vi "main.vi"() -> ()   [LabVIEW 2021]
uses:
  <vilib>/xnet/xnet.llb/XNET Frame CAN.ctl
  <vilib>/xnet/xnet.llb/XNET Frame Type CAN.ctl
  General Purpose/measurements.ctl
  General Purpose/measurements_SC.ctl
  active-front-ends/Time-sync/time_sync/TypeDef/Synch_shift--cluster.ctl
  <vilib>/Platform/TimedLoop/XDataNode/timing_clust.ctl
  <vilib>/Platform/TimedLoop/XDataNode/nitl_modes.ctl
  <vilib>/Platform/TimedLoop/XDataNode/wakeup.ctl
  communication/PVemulator_Central.ctl
  communication/PVemulator_Central_Info.ctl
  communication/PVemulator_Central_Data.ctl
  communication/SC_references.ctl
  central data acquisition/MeteoBoxCentral.ctl
  central data acquisition/MeteoBoxCentral_Info.ctl
  central data acquisition/MeteoBoxCentral_Data.ctl
  <vilib>/xnet/xnet.llb/XNET Write (Frame CAN).vi
  <vilib>/xnet/xnet.llb/XNET Read (Frame CAN).vi
  <vilib>/Platform/TimedLoop/XDataNode/XDataNode.xnode
  <vilib>/Platform/TimedLoop/XDataNode/XDNodeRunTimeDep.lvlib
  <userlib>/_OpenG.lib/boolean/boolean.llb/openg_boolean__ogtk.lvlib
panel:
  out "Period":i64
  out "follow":timestamp
  out "form":timestamp
  out "time_sc":timestamp
  out "start following SC pre":bool
  out "forming?":bool
  out "Ready SC":bool
  out "OFF SC":bool
  out "V slider 31":dbl(slide) caption="V-i" max=-10.0 scale=0.0..100.0 scale format="%#_4g"
  in  "SEND sp SC":bool
  in  "Start following SC":bool
  in  "Start forming SC":bool
  in  "Vdc SC":dbl
  out "Synch Monitor":string[][](table)
  in  "Loop Time":u32=125
  out "Error out":errorcluster
  in  "Timeout [ms]":i32=3000
  out "Offset from TR (ns)":dbl
  out "Status Out":T1
  out "ON SC":bool
  out "state SC":u16
  out "measurements SuperCap":T2
  out "V slider 29":dbl(slide) caption="V-i" max=-10.0 scale=650.0..780.0 scale format="%#_4g"
  out "V slider 30":dbl(slide) caption="V-i" max=-10.0 scale=650.0..780.0 scale format="%#_4g"
  out "kW":dbl caption="Numeric" format="%#.3g"
  in  "Pdc SC":dbl
  in  "Shutdwn SC":bool
  in  "Use METEO":bool
  out "Temps":dbl[](array[numeric])
  out "GHIs":dbl[](array[numeric])
  out "Meteo.Tair":dbl
  out "Meteo.GHI":dbl
  in  "Update setpoints":bool
  out "V slider 28":dbl(slide) caption="V-i" max=-10.0 scale=650.0..780.0 scale format="%#_4g"
  out "V slider 27":dbl(slide) caption="V-i" max=-10.0 scale=650.0..780.0 scale format="%#_4g"
  out "V slider 26":dbl(slide) caption="V-i" max=-10.0 scale=650.0..780.0 scale format="%#_4g"
  out "V slider 25":dbl(slide) caption="V-i" max=-10.0 scale=650.0..780.0 scale format="%#_4g"
  out "V slider 24":dbl(slide) caption="V-i" max=-10.0 scale=650.0..780.0 scale format="%#_4g"
  out "V slider 23":dbl(slide) caption="V-i" max=-10.0 scale=650.0..780.0 scale format="%#_4g"
  out "V slider 22":dbl(slide) caption="V-i" max=-10.0 scale=650.0..780.0 scale format="%#_4g"
  out "V slider 21":dbl(slide) caption="V-i" max=-10.0 scale=650.0..780.0 scale format="%#_4g"
  in  "P 4":dbl
  in  "P 3":dbl
  in  "P 2":dbl
  out "state 4":u16
  out "state 3":u16
  out "state 2":u16
  out "state 1":u16
  out "kW":dbl caption="Numeric" format="%#.3g"
  out "kW":dbl caption="Numeric" format="%#.3g"
  out "kW":dbl caption="Numeric" format="%#.3g"
  out "kW":dbl caption="Numeric" format="%#.3g"
  in  "P 1":dbl
  out "current time":timestamp
  in  "measurements":T3
  out "CAN OUT":T4 {"payload" format="%x"; "timestamp" format="%<%.7X\n%x>T"; "type" items=["CAN Data"=0, "CAN Remote"=1, "CAN Bus Error"=2, "CAN 2.0 Data"=8, "CAN FD Data"=16, "CAN FD+BRS Data"=24, "J1939 Data"=192, "Delay"=224, "Log Trigger"=225, "Start Trigger"=226]; "identifier" format="%x"}
  in  "EnablePR 4":bool
  in  "EnablePR 3":bool
  in  "EnablePR 2":bool
  in  "EnablePR 1":bool
  in  "main stop":bool
  in  "DCLinkOK  4":bool
  in  "PowerEnable 4":bool
  in  "ErrAck 4":bool
  in  "Shutdwn 4":bool
  in  "DCLinkOK  3":bool
  in  "PowerEnable 3":bool
  in  "ErrAck 3":bool
  in  "Shutdwn 3":bool
  in  "DCLinkOK 2":bool
  in  "PowerEnable 2":bool
  in  "ErrAck 2":bool
  in  "Shutdwn 2":bool
  out "OFF 4":bool
  out "ON 4":bool
  out "Ready 4":bool
  out "OFF 3":bool
  out "ON 3":bool
  out "Ready 3":bool
  out "OFF 2":bool
  out "ON 2":bool
  out "Ready 2":bool
  out "error out":errorcluster
  out "OFF 1":bool
  out "ON 1":bool
  out "Ready 1":bool
  out "CAN IN":T4 {"payload" format="%x"; "timestamp" format="%<%.7X\n%x>T"; "type" items=["CAN Data"=0, "CAN Remote"=1, "CAN Bus Error"=2, "CAN 2.0 Data"=8, "CAN FD Data"=16, "CAN FD+BRS Data"=24, "J1939 Data"=192, "Delay"=224, "Log Trigger"=225, "Start Trigger"=226]; "identifier" format="%x"}
  in  "CAN [ms]":i64=1
  out "CAN with Conv":bool
  out "Measurements":bool
  in  "Shutdwn 1":bool
  in  "ErrAck 1":bool
  in  "PowerEnable 1":bool
  in  "DCLinkOK 1":bool
  # "PV emulators 1-4"
  # "B22"
  # "DC"
  # "PV 4"
  # "DC"
  # "B21"
  # "DC"
  # "PV 3"
  # "DC"
  # "B20"
  # "DC"
  # "PV 2"
  # "DC"
  # "B19"
  # "1"
  # "DC"
  # "2"
  # "PV 1"
  # "3"
  # "DC"
  # "DC"
  # "SC"
  # "DC"
  # "SOC"
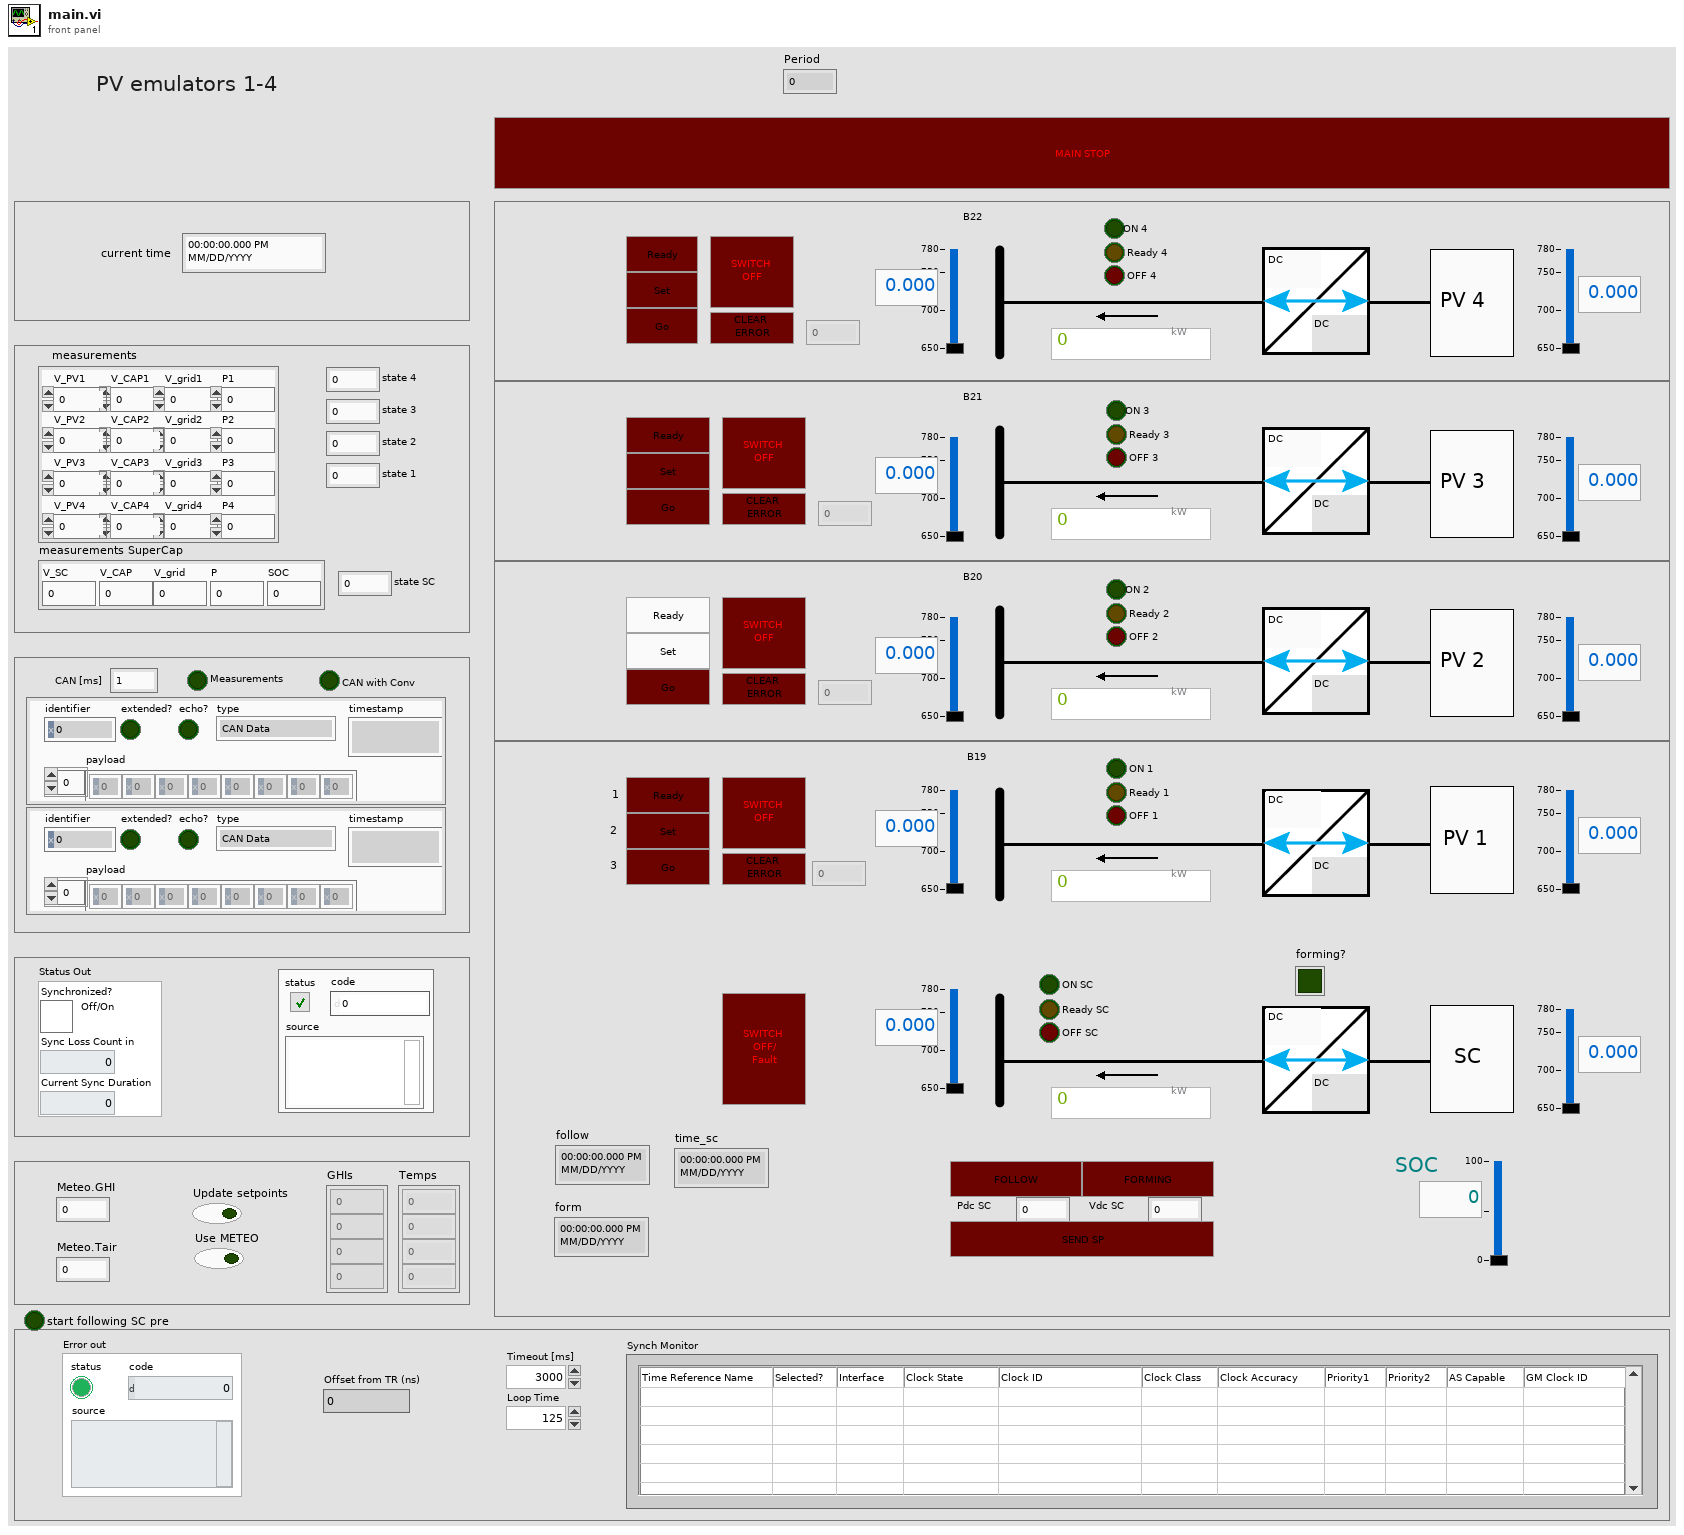
[diagram p1: front panel]
types:
  T1 = typedef "Synch_shift--cluster.ctl" = cluster{"Synchronized?":bool, "Sync Loss Count in":u32, "Current Sync Duration":u32}
  T2 = typedef "measurements_SC.ctl" = cluster{"V_SC":dbl, "V_CAP":dbl, "V_grid":dbl, "P":dbl, "SOC":dbl}
  T3 = typedef "measurements.ctl" = cluster{"V_PV1":dbl, "V_CAP1":dbl, "V_PV2":dbl, "V_CAP2":dbl, "V_grid2":dbl, "V_PV3":dbl, "V_CAP3":dbl, "V_grid3":dbl, "V_PV4":dbl, "V_CAP4":dbl, "V_grid4":dbl, "V_grid1":dbl, "P1":dbl, "P2":dbl, "P3":dbl, "P4":dbl}
  T4 = typedef "XNET Frame CAN.ctl" = cluster{"timestamp":timestamp, "payload":u8[], "identifier":u32, "type":T5, "extended?":bool, "echo?":bool}
  T5 = typedef "XNET Frame Type CAN.ctl" = u8
  T6 = cluster{"Frame In":refnum<k21>, "Frame Out":refnum<k21>}
  T7 = typedef "XDNodeRunTimeDep.lvlib/timing_clust.ctl" = cluster{"Expected End [f-1]":u64, "Actual End [f-1]":u64, "Finished Late? [f-1]":bool, "Expected End [i-1]":u64, "Actual End [i-1]":u64, "Finished Late? [i-1]":bool, "Expected Start [i]":u64, "Actual Start [i]":u64, "Expected Start [f]":u64, "Actual Start [f]":u64, "Source Name":string, "Structure Name":string, "Period":i64, "Deadline":i64, "Offset":i64, "Start":i64, "Priority":i32, "Timeout":i32, "Mode":T8, "Wakeup Reason":T9, "Error":errorcluster, "Source Type":string, "Secondary Source Type":string, "Global End Time":u64, "Global Start Time":u64, "Frame Duration":u64, "Iteration Duration":u64, "Assigned CPU":i32, "I/O Scan Engine Mode":u32}
  T8 = typedef "XDNodeRunTimeDep.lvlib/nitl_modes.ctl" = enum32{"No Change", "Process missed periods, maintain original phase", "Discard missed periods, maintain original phase", "Process missed periods, ignore original phase", "Discard missed periods, ignore original phase"}
  T9 = typedef "XDNodeRunTimeDep.lvlib/wakeup.ctl" = enum32{"Normal", "Aborted", "Asynchronous wakeup", "Timing source error", "Timed loop error", "Timeout"}
  T10 = typedef "MeteoBoxCentral.ctl" = cluster{"Info":T11, "Data":T12}
  T11 = typedef "MeteoBoxCentral_Info.ctl" = cluster{"Resource":string, "Problem":bool, "Timestamp":dbl}
  T12 = typedef "MeteoBoxCentral_Data.ctl" = cluster{"GI":dbl, "GHI":dbl, "GVI":dbl, "Tair":dbl, "Tcell":dbl, "Global_Total_Irr":dbl, "Diffused_Irr":dbl}
  T13 = typedef "PVemulator_Central.ctl" = cluster{"Info":T14, "Data":T15}
  T14 = typedef "PVemulator_Central_Info.ctl" = cluster{"Resource":string, "Problem":bool, "Timestamp":dbl}
  T15 = typedef "PVemulator_Central_Data.ctl" = cluster{"Status 1":bool, "Status 2":bool, "measurements":T3, "Status 3":bool, "Status 4":bool, "measurements SC":T2, "Status SC":bool, "Forming/Following":bool, "Start forming":bool, "SC references":T16, "Start following":bool}
  T16 = typedef "SC_references.ctl" = cluster{"Vdc":dbl, "Pdc":dbl}
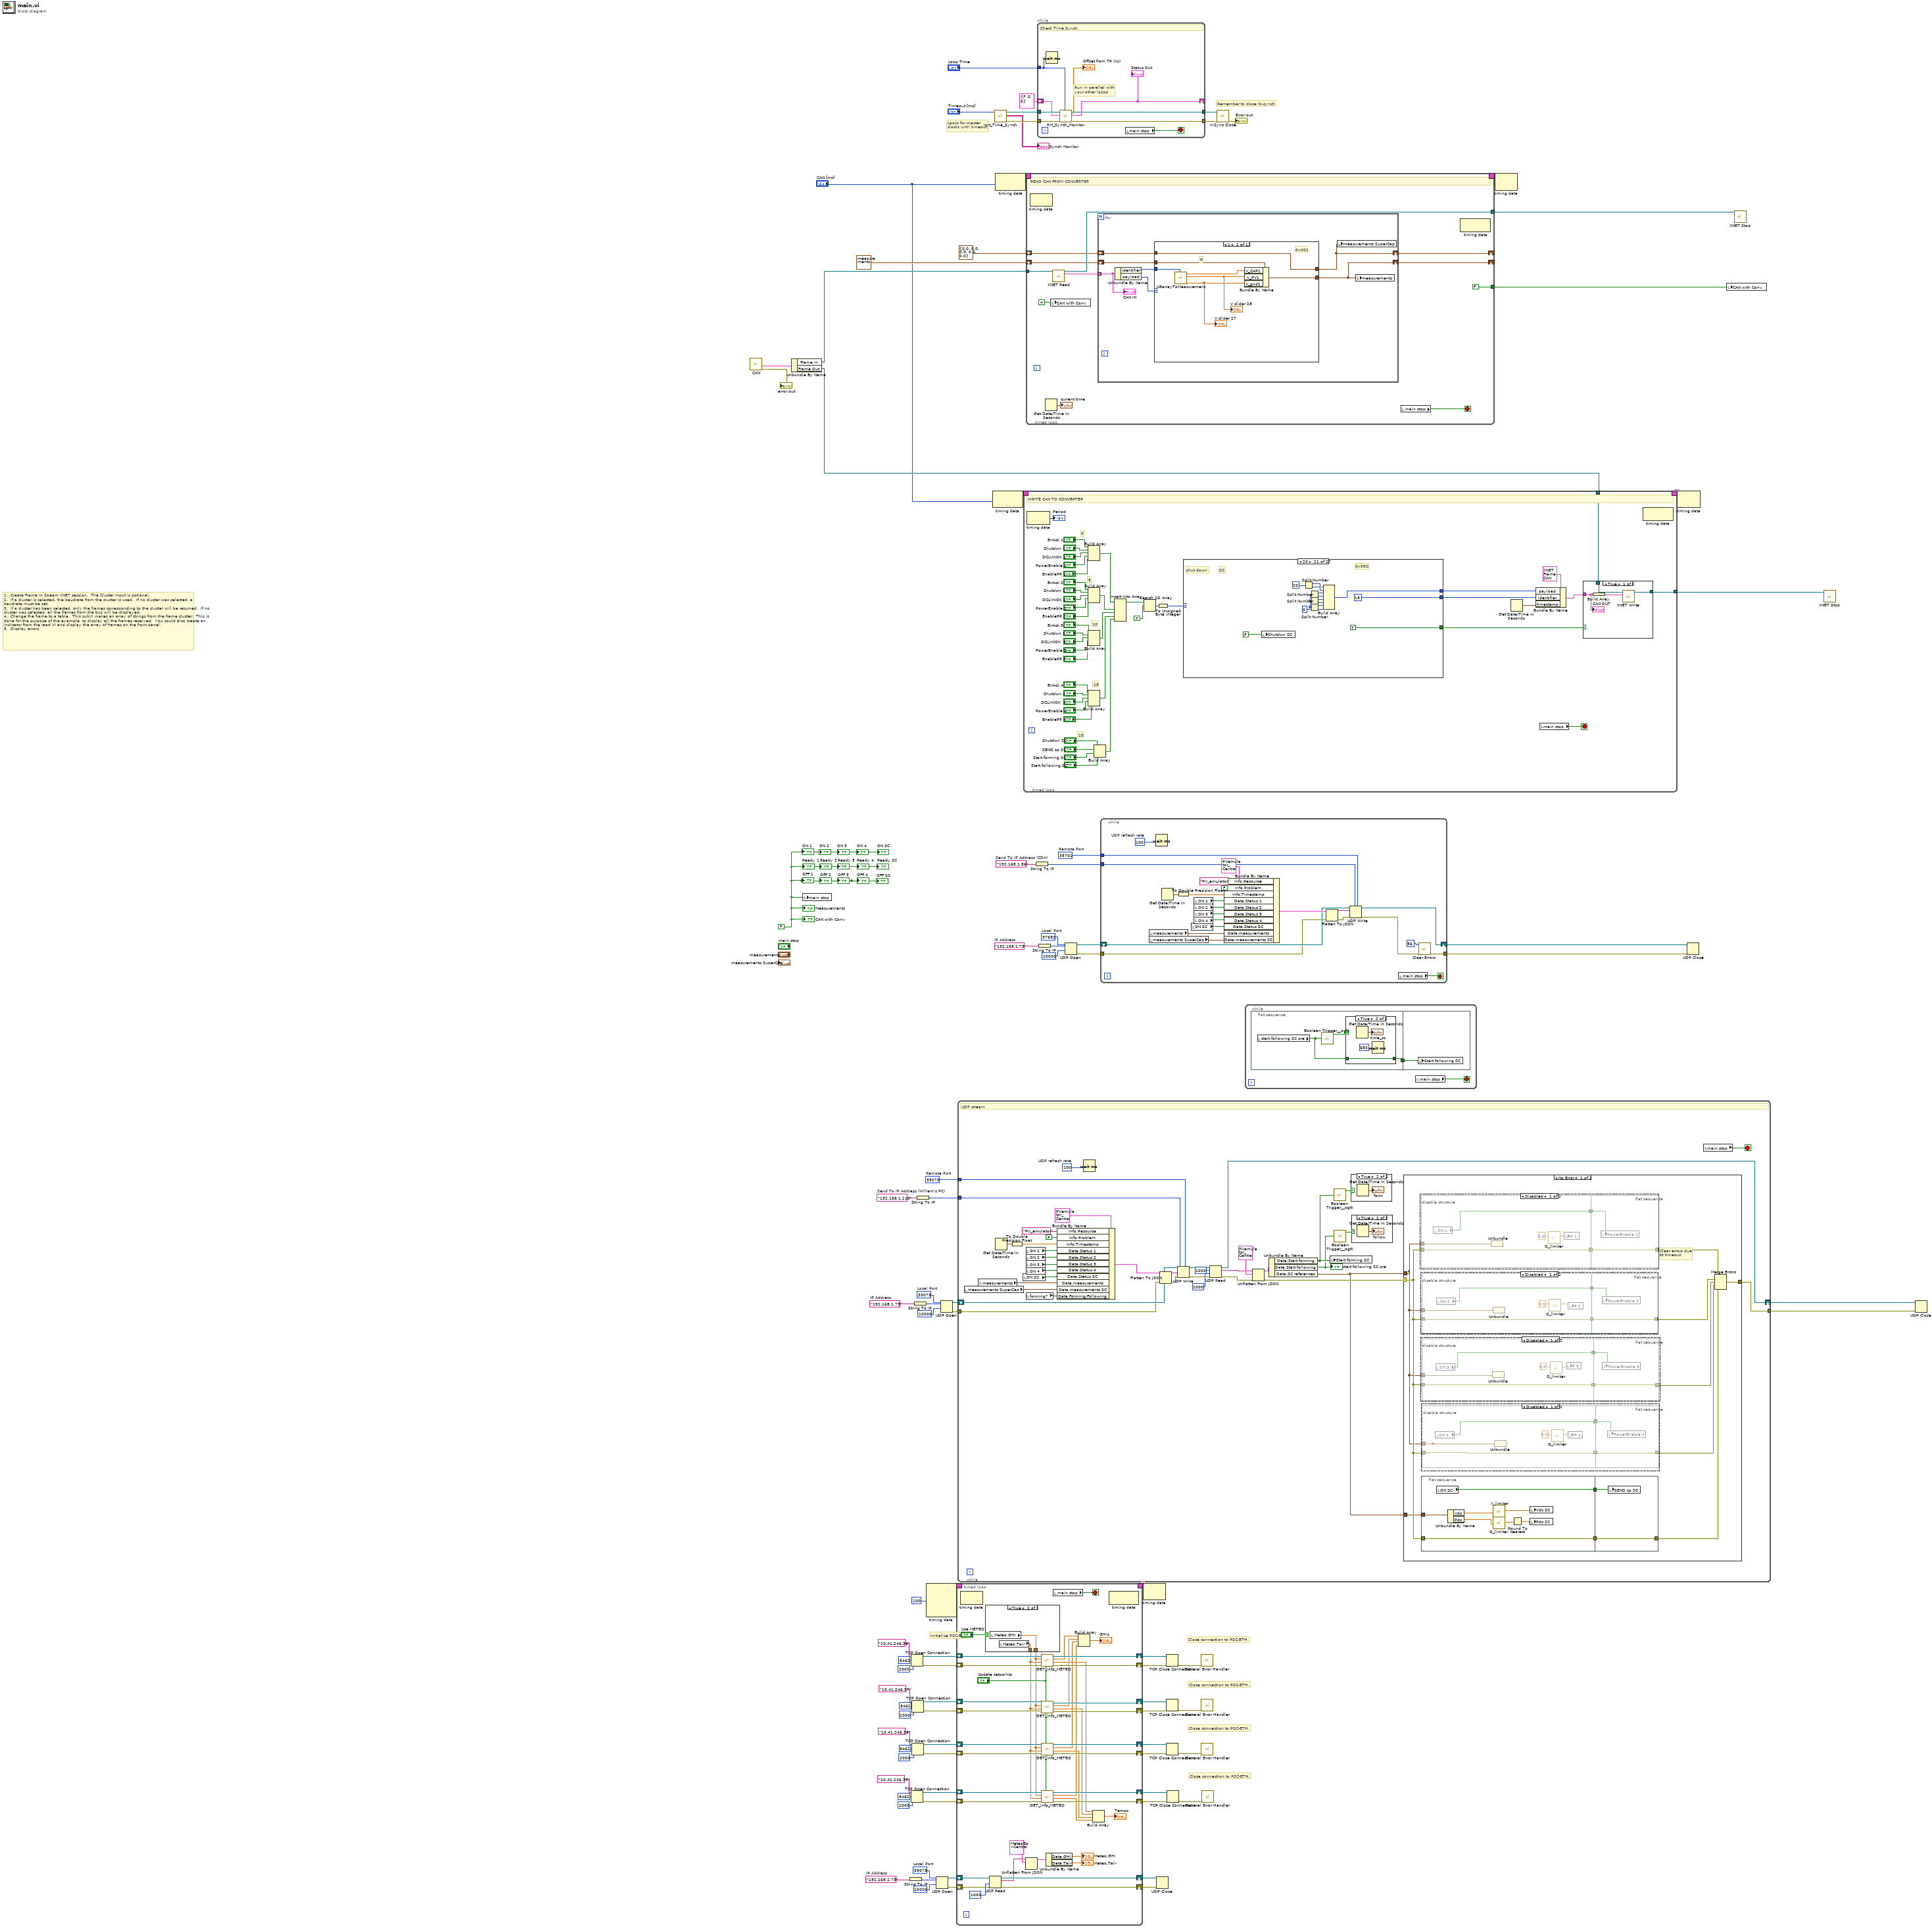
[diagram p0: block diagram]
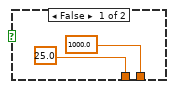
[diagram p10: hidden frame]
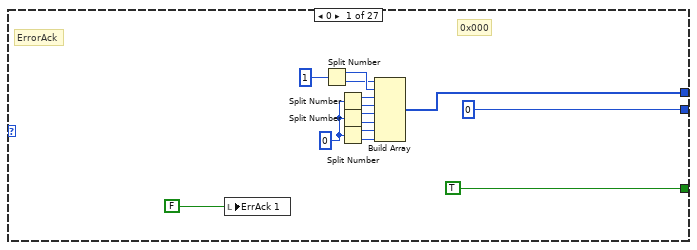
[diagram p12: hidden frame]
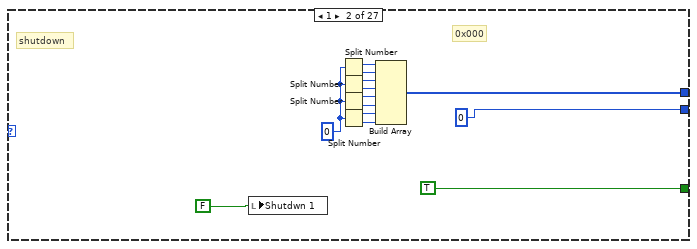
[diagram p13: hidden frame]
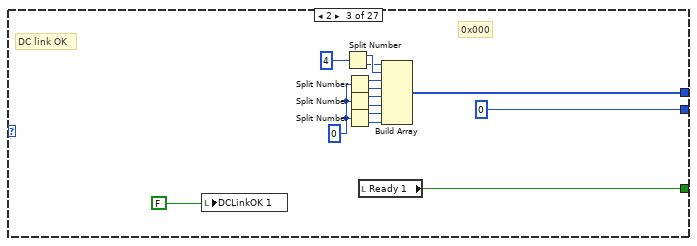
[diagram p14: hidden frame]
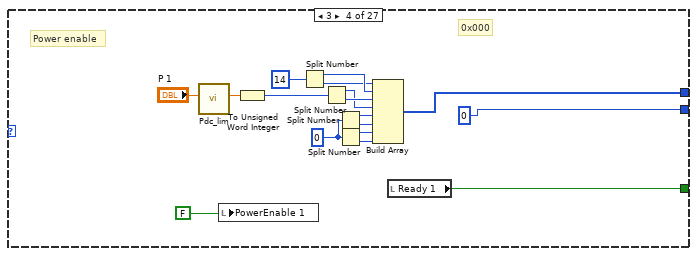
[diagram p15: hidden frame]
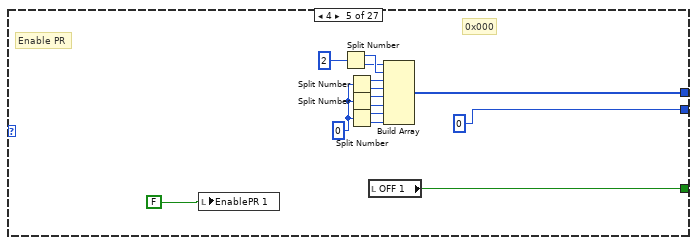
[diagram p16: hidden frame]
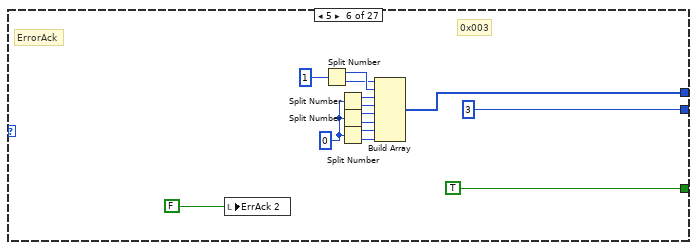
[diagram p17: hidden frame]
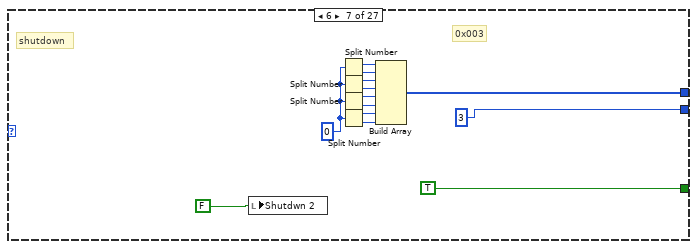
[diagram p18: hidden frame]
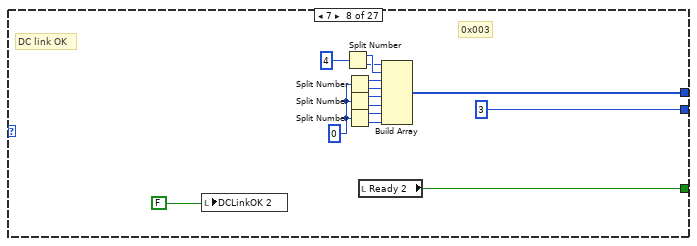
[diagram p19: hidden frame]
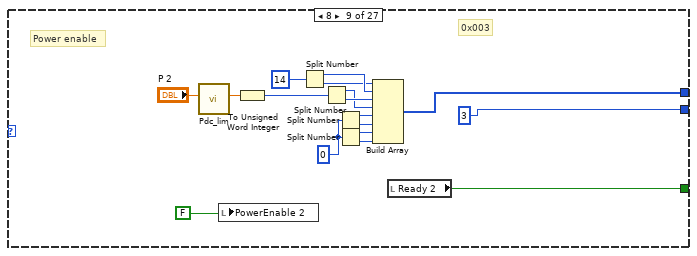
[diagram p20: hidden frame]
diagram:
  w12 = u16 35073  # Remote Port
  w14 = "192.168.1.210"  # Send To IP Address (Willem's PC)
  w18 = u16 33073  # Local Port
  w19 = "192.168.1.73"  # IP Address
  w59 = u16 39073  # Local Port
  w60 = "192.168.1.73"  # IP Address
  w77 = u16 37692  # Local Port
  w78 = "192.168.1.73"  # IP Address
  w8 = u16 35701  # Remote Port
  w76 = "192.168.1.86"  # Send To IP Address (CDA)
  w2 = FALSE
  # "Remember to close NI-synch"
  # "Looks for master \nclocks until timeout"
  # "Close connection to PSC-ETH."
  # "Close connection to PSC-ETH."
  # "Close connection to PSC-ETH."
  # "Close connection to PSC-ETH."
  # "Initialize PSC-ETH"
  # "1.  Create Frame In Stream XNET session.  The Cluster input is optional.  \n2.  If a cluster is selected, the baudrate from the cluster is used.  If no cluster was selected, a baudrate must be set.\n3.  If a cluster has been selected, only the frames corresponding to the cluster will be returned.  If no cluster was selected, all the frames from the bus will be displayed.\n4.  Change the frame to a table.  This subVI makes an array of strings from the frame cluster.  This is done for the purpose of the example, to display all the frames received.  You could also create an indicator from the read VI and display the array of frames on the front panel. \n5.  Display errors."
  n1 = call "CAN.vi"() -> ("error out"=→"error out":errorcluster, "CAN"=w74:T6)  [unwired: 9 in, 1 out]
  n2 = Unbundle By Name(w74) -> ("Frame In"=w83:refnum<k21>, "Frame Out"=w86:refnum<k21>)
  n3 = local write "main stop"(w2) -> ()
  n4 = String To IP(1:w60) -> (0:w61:u32)
  n5 = TCP Open Connection(address="10.41.246.39", remote port or service name=u16 8462 ("remote port"), timeout ms (60000)=2000) -> (connection ID=w44:refnum<k5>, error out=w43:errorcluster)  [unwired: 2 in]
  n6 = TCP Open Connection(address="10.41.246.36", remote port or service name=u16 8462 ("remote port"), timeout ms (60000)=2000) -> (connection ID=w66:refnum<k5>, error out=w65:errorcluster)  [unwired: 2 in]
  n7 = TCP Open Connection(address="10.41.246.38", remote port or service name=u16 8462 ("remote port"), timeout ms (60000)=2000) -> (connection ID=w46:refnum<k5>, error out=w45:errorcluster)  [unwired: 2 in]
  n8 = TCP Open Connection(address="10.41.246.37", remote port or service name=u16 8462 ("remote port"), timeout ms (60000)=2000) -> (connection ID=w48:refnum<k5>, error out=w47:errorcluster)  [unwired: 2 in]
  n9 = String To IP(1:w19) -> (0:w20:u32)
  n10 = String To IP(1:w14) -> (0:w13:u32)
  n11 = node-c288(i64 100 ("Period")) -> (w72:T7)  [unwired: 3 in]
  n12 = UDP Open(7:w61, 9:10000 ("timeout ms (25000)"), 11:w59) -> (port=w33:refnum<k16>, 0:w32:errorcluster)  [unwired: 2 in, 1 out]
  n13 = UDP Open(7:w20, 9:10000 ("timeout ms (25000)"), 11:w18) -> (port=w15:refnum<k16>, 0:w16:errorcluster)  [unwired: 2 in, 1 out]
  n14 = timed-loop {
    timing: w72 -> [_]
    timing-out: [_] -> w71
    shift-right: [w127] -> w63
    shift-left: w66 -> [w129]
    shift-right: [w126] -> w62
    shift-left: w65 -> [w128]
    shift-right: [w118] -> w38
    shift-left: w47 -> [w124]
    shift-right: [w119] -> w39
    shift-left: w48 -> [w125]
    shift-right: [w117] -> w37
    shift-left: w46 -> [w123]
    shift-right: [w116] -> w36
    shift-left: w45 -> [w122]
    shift-right: [w115] -> w35
    shift-left: w44 -> [w121]
    shift-right: [w114] -> w34
    shift-left: w43 -> [w120]
    shift-right: [w92] -> w31
    shift-left: w33 -> [w94]
    shift-right: [w91] -> w30
    shift-left: w32 -> [w93]
    stop <- w130 stop-if-true
    n15 = node-c288() -> ()  [unwired: 1 in, 1 out]
    n16 = case shown="True" "Use METEO" {
      tunnel: [1000.0 ("Meteo.GHI") w133] -> w112
      tunnel: [25.0 ("Meteo.Tair") w134] -> w111
      frame False {
      }
      frame True {
        n17 = local read "Meteo.GHI"() -> (w133:dbl)
        n18 = local read "Meteo.Tair"() -> (w134:dbl)
      }
    }
    n19 = UDP Read(connection ID=w94, timeout ms (25000)=1000, 8:w93) -> (data out=w96:string, error out=w91:errorcluster, 3:w92:refnum<k16>)  [unwired: 1 in, 2 out]
    n20 = Unflatten From JSON(JSON string=w96, type and defaults=T10 {"Info"={"Resource"="MeteoBox", "Problem"=FALSE, "Timestamp"=0.0}, "Data"={"GI"=0.0, "GHI"=0.0, "GVI"=0.0, "Tair"=0.0, "Tcell"=0.0, "Global_Total_Irr"=0.0, "Diffused_Irr"=0.0}} ("Cluster")) -> (value=w98:T10)  [unwired: 5 in, 1 out]
    n21 = call "GET_info_METEO.vi"("Update GHI"="Update setpoints", "error in"=w128, "set Temp"=w111, "set GHI"=w112, "connection ID in"=w129) -> ("error out"=w126:errorcluster, "read Temp"=w102:dbl, "read GHI"=w110:dbl, "connection ID out"=w127:refnum<k5>)  [unwired: 3 in]
    n22 = call "GET_info_METEO.vi"("Update GHI"="Update setpoints", "error in"=w124, "set Temp"=w111, "set GHI"=w112, "connection ID in"=w125) -> ("error out"=w118:errorcluster, "read Temp"=w103:dbl, "read GHI"=w109:dbl, "connection ID out"=w119:refnum<k5>)  [unwired: 3 in]
    n23 = call "GET_info_METEO.vi"("Update GHI"="Update setpoints", "error in"=w122, "set Temp"=w111, "set GHI"=w112, "connection ID in"=w123) -> ("error out"=w116:errorcluster, "read Temp"=w104:dbl, "read GHI"=w108:dbl, "connection ID out"=w117:refnum<k5>)  [unwired: 3 in]
    n24 = call "GET_info_METEO.vi"("Update GHI"="Update setpoints", "error in"=w120, "set Temp"=w111, "set GHI"=w112, "connection ID in"=w121) -> ("error out"=w114:errorcluster, "read Temp"=w105:dbl, "read GHI"=w107:dbl, "connection ID out"=w115:refnum<k5>)  [unwired: 3 in]
    n25 = Unbundle By Name(w98) -> ("Data.GHI"=→"Meteo.GHI":dbl, "Data.Tair"=→"Meteo.Tair":dbl)
    n26 = local read "main stop"() -> (w130:bool)
    n27 = Build Array(w110, w109, w108, w107) -> (→"GHIs":dbl[])
    n28 = Build Array(w102, w103, w104, w105) -> (→"Temps":dbl[])
    n29 = node-c288() -> ()  [unwired: 1 in, 1 out]
  }
  n30 = while {
    tunnel: w16 -> [w157]
    tunnel: w13 -> [w171]
    tunnel: w12 -> [w170]
    shift-right: [w167] -> w11
    shift-left: w15 -> [w172]
    tunnel: [w148] -> w3
    stop <- w174 stop-if-true
    w166 = u32 100  # UDP refresh rate
    # "Clear errors due\nto timeout"
    # "UDP stream"
    n31 = local read "measurements SuperCap"() -> (w151:T2)
    n32 = local read "measurements"() -> (w150:T3)
    n33 = Get Date/Time In Seconds() -> (seconds since 1Jan1904=w164:timestamp)
    n34 = To Double Precision Float(number=w164) -> (double precision float=w165:dbl)
    n35 = local read "ON SC"() -> (w152:bool)
    n36 = local read "ON 1"() -> (w156:bool)
    n37 = local read "ON 2"() -> (w155:bool)
    n38 = local read "ON 3"() -> (w154:bool)
    n39 = local read "ON 4"() -> (w153:bool)
    n40 = local read "forming?"() -> (w141:bool)
    n41 = Bundle By Name(cluster=T13 {"Info"={"Resource"="PV_emulator", "Problem"=FALSE, "Timestamp"=0.0}, "Data"={"Status 1"=FALSE, "Status 2"=FALSE, "measurements"={"V_PV1"=0.0, "V_CAP1"=0.0, "V_PV2"=0.0, "V_CAP2"=0.0, "V_grid2"=0.0, "V_PV3"=0.0, "V_CAP3"=0.0, "V_grid3"=0.0, "V_PV4"=0.0, "V_CAP4"=0.0, "V_grid4"=0.0, "V_grid1"=0.0, "P1"=0.0, "P2"=0.0, "P3"=0.0, "P4"=0.0}, "Status 3"=FALSE, "Status 4"=FALSE, "measurements SC"={"V_SC"=0.0, "V_CAP"=0.0, "V_grid"=0.0, "P"=0.0, "SOC"=0.0}, "Status SC"=FALSE, "Forming/Following"=FALSE, "Start forming"=FALSE, "SC references"={"Vdc"=0.0, "Pdc"=0.0}, "Start following"=FALSE}} ("Cluster"), "Info.Resource"="PV_emulator", "Info.Problem"=FALSE, "Info.Timestamp"=w165, "Data.Status 1"=w156, "Data.Status 2"=w155, "Data.Status 3"=w154, "Data.Status 4"=w153, "Data.Status SC"=w152, "Data.measurements"=w150, "Data.measurements SC"=w151, "Data.Forming/Following"=w141) -> (w159:T13)
    n42 = Wait (ms)(milliseconds to wait=w166) -> ()  [unwired: 1 out]
    n43 = Flatten To JSON(anything=w159, error in (no error)=w157) -> (JSON string=w163:string, 11:w158:errorcluster)  [unwired: 1 in]
    n44 = UDP Write(address=w171, port or service name=w170, connection ID=w172, data in=w163, 8:w158) -> (error out=w168:errorcluster, 3:w169:refnum<k16>)  [unwired: 1 in]
    n45 = UDP Read(connection ID=w169, max size (548)=1000, timeout ms (25000)=1000, 8:w168) -> (data out=w145:string, error out=w147:errorcluster, 3:w167:refnum<k16>)  [unwired: 2 out]
    n46 = Unflatten From JSON(JSON string=w145, type and defaults=T13 {"Info"={"Resource"="PV_emulator", "Problem"=FALSE, "Timestamp"=0.0}, "Data"={"Status 1"=FALSE, "Status 2"=FALSE, "measurements"={"V_PV1"=0.0, "V_CAP1"=0.0, "V_PV2"=0.0, "V_CAP2"=0.0, "V_grid2"=0.0, "V_PV3"=0.0, "V_CAP3"=0.0, "V_grid3"=0.0, "V_PV4"=0.0, "V_CAP4"=0.0, "V_grid4"=0.0, "V_grid1"=0.0, "P1"=0.0, "P2"=0.0, "P3"=0.0, "P4"=0.0}, "Status 3"=FALSE, "Status 4"=FALSE, "measurements SC"={"V_SC"=0.0, "V_CAP"=0.0, "V_grid"=0.0, "P"=0.0, "SOC"=0.0}, "Status SC"=FALSE, "Forming/Following"=FALSE, "Start forming"=FALSE, "SC references"={"Vdc"=0.0, "Pdc"=0.0}, "Start following"=FALSE}} ("Cluster"), error in (no error)=w147) -> (value=w143:T13, error out=w146:errorcluster)  [unwired: 4 in]
    n47 = Unbundle By Name(w143) -> ("Data.Start forming"=w138:bool, "Data.Start following"=w137:bool, "Data.SC references"=w142:T16)
    "start following SC pre" <- w137
    n48 = local write "Start forming SC"(w138) -> ()
    n49 = call <userlib>:"Boolean Trigger__ogtk.vi"("Boolean Input"=w138) -> ("Rising Edge"=w140:bool)  [unwired: 1 in, 1 out]
    n50 = call <userlib>:"Boolean Trigger__ogtk.vi"("Boolean Input"=w137) -> ("Rising Edge"=w139:bool)  [unwired: 1 in, 1 out]
    n51 = case shown="True" w140 {
      frame False {
      }
      frame True {
        n52 = Get Date/Time In Seconds() -> (seconds since 1Jan1904=→"form":timestamp)
      }
    }
    n53 = case shown="True" w139 {
      frame False {
      }
      frame True {
        n54 = Get Date/Time In Seconds() -> (seconds since 1Jan1904=→"follow":timestamp)
      }
    }
    n55 = case shown="No Error" w146 {
      selector: w146 -> [w182 w246]
      tunnel: [w187 w246] -> w148
      tunnel: w142 -> [w178 _]
      tunnel: w142 -> [w177 _]
      frame No Error {
        n56 = disable-structure shown="Disabled" {
          disable-tunnel: [w226 _] -> w186
          disable-tunnel: w182 -> [w225 _]
          disable-tunnel: w177 -> [w224 _]
          frame Disabled {
            n57 = flat-sequence {
              tunnel: w225 -> [w233]
              tunnel: [w233] -> w228
              tunnel: [w232] -> w227
              tunnel: w224 -> [w231]
              tunnel: w228 -> [w235]
              tunnel: [w235] -> w226
              tunnel: w227 -> [w234]
              frame #0 {
                n58 = local read "ON 1"() -> (w232:bool)
                n59 = Unbundle(w231) -> ()  [unwired: 2 out]
                n60 = call "Q_limiter.vi"("IN Q"=0.0) -> ("OUT Q"=w230:dbl)  [unwired: 10 in]
                n61 = local write "P 1"(w230) -> ()
              }
              frame #1 {
                n62 = local write "PowerEnable 1"(w234) -> ()
              }
            }
          }
          frame Enabled {
          }
        }
        n63 = disable-structure shown="Disabled" {
          disable-tunnel: [w214 _] -> w184
          disable-tunnel: w182 -> [w213 _]
          disable-tunnel: w177 -> [w212 _]
          frame Disabled {
            n64 = flat-sequence {
              tunnel: w213 -> [w221]
              tunnel: w212 -> [w220]
              tunnel: [w221] -> w216
              tunnel: [w219] -> w215
              tunnel: [w223] -> w214
              tunnel: w216 -> [w223]
              tunnel: w215 -> [w222]
              frame #0 {
                n65 = local read "ON 2"() -> (w219:bool)
                n66 = Unbundle(w220) -> ()  [unwired: 2 out]
                n67 = call "Q_limiter.vi"("IN Q"=0.0) -> ("OUT Q"=w218:dbl)  [unwired: 10 in]
                n68 = local write "P 2"(w218) -> ()
              }
              frame #1 {
                n69 = local write "PowerEnable 2"(w222) -> ()
              }
            }
          }
          frame Enabled {
          }
        }
        n70 = disable-structure shown="Disabled" {
          disable-tunnel: [w202 _] -> w185
          disable-tunnel: w182 -> [w201 _]
          disable-tunnel: w177 -> [w200 _]
          frame Disabled {
            n71 = flat-sequence {
              tunnel: w201 -> [w209]
              tunnel: w200 -> [w208]
              tunnel: [w209] -> w204
              tunnel: [w207] -> w203
              tunnel: [w211] -> w202
              tunnel: w204 -> [w211]
              tunnel: w203 -> [w210]
              frame #0 {
                n72 = local read "ON 3"() -> (w207:bool)
                n73 = Unbundle(w208) -> ()  [unwired: 2 out]
                n74 = call "Q_limiter.vi"("IN Q"=0.0) -> ("OUT Q"=w206:dbl)  [unwired: 10 in]
                n75 = local write "P 3"(w206) -> ()
              }
              frame #1 {
                n76 = local write "PowerEnable 3"(w210) -> ()
              }
            }
          }
          frame Enabled {
          }
        }
        n77 = disable-structure shown="Disabled" {
          disable-tunnel: w182 -> [w190 _]
          disable-tunnel: [w189 _] -> w180
          disable-tunnel: w177 -> [w188 _]
          frame Disabled {
            n78 = flat-sequence {
              tunnel: w190 -> [w197]
              tunnel: [w196] -> _
              tunnel: w188 -> [w196]
              tunnel: [w197] -> w192
              tunnel: [w195] -> w191
              tunnel: [w199] -> w189
              tunnel: w192 -> [w199]
              tunnel: w191 -> [w198]
              frame #0 {
                n79 = local read "ON 4"() -> (w195:bool)
                n80 = Unbundle(w196) -> ()  [unwired: 2 out]
                n81 = call "Q_limiter.vi"("IN Q"=0.0) -> ("OUT Q"=w194:dbl)  [unwired: 10 in]
                n82 = local write "P 4"(w194) -> ()
              }
              frame #1 {
                n83 = local write "PowerEnable 4"(w198) -> ()
              }
            }
          }
          frame Enabled {
          }
        }
        n84 = flat-sequence {
          tunnel: [w236] -> w183
          tunnel: w182 -> [w240]
          tunnel: [w240] -> w181
          tunnel: w178 -> [w241]
          tunnel: w183 -> [w245]
          tunnel: [w244] -> w179
          tunnel: w181 -> [w244]
          frame #0 {
            n85 = local read "ON SC"() -> (w236:bool)
            n86 = Unbundle By Name(w241) -> ("Vdc"=w243:dbl, "Pdc"=w242:dbl)
            n87 = call "V_limiter.vi"("IN Q"=w243) -> ("OUT Q"=w237:dbl)  [unwired: 10 in]
            n88 = call "Q_limiter.vi"("IN Q"=w242) -> ("OUT Q"=w239:dbl)  [unwired: 10 in]
            n89 = Round To Nearest(number=w239) -> (nearest integer value=w238:dbl)
            n90 = local write "Vdc SC"(w237) -> ()
            n91 = local write "Pdc SC"(w238) -> ()
          }
          frame #1 {
            n92 = local write "SEND sp SC"(w245) -> ()
          }
        }
        n93 = Merge Errors(w186, w184, w185, w180, w179) -> (w187:errorcluster)
      }
      frame Error {
      }
    }
    n94 = local read "main stop"() -> (w174:bool)
  }
  n95 = node-c288("CAN [ms]") -> (w81:T7)
  n96 = call "Init_Time_Synch.vi"("Timeout [ms]"="Timeout [ms]") -> ("Error out"=w28:errorcluster, "Synch Monitor"=→"Synch Monitor":string[][], "Synch Out"=w26:refnum<k15>)  [unwired: 7 in, 1 out]
  n97 = node-c288("CAN [ms]") -> (w85:T7)
  n98 = timed-loop {
    tunnel: w86 -> [w285]
    tunnel: [w284] -> w88
    timing: w81 -> [_]
    timing-out: [_] -> w80
    stop <- w283 stop-if-true
    # "15"
    # "10"
    # "5"
    # "0"
    # "20"
    # "WRITE CAN TO CONVERTER"
    n99 = node-c288() -> (→"Period":i64)  [unwired: 1 in]
    n100 = Build Array("ErrAck 1", "Shutdwn 1", "DCLinkOK 1", "PowerEnable 1", "EnablePR 1") -> (w264:bool[])
    n101 = Build Array("ErrAck 2", "Shutdwn 2", "DCLinkOK 2", "PowerEnable 2", "EnablePR 2") -> (w263:bool[])
    n102 = Build Array("ErrAck 3", "Shutdwn 3", "DCLinkOK  3", "PowerEnable 3", "EnablePR 3") -> (w262:bool[])
    n103 = Build Array("ErrAck 4", "Shutdwn 4", "DCLinkOK  4", "PowerEnable 4", "EnablePR 4") -> (w261:bool[])
    n104 = Build Array("Shutdwn SC", "SEND sp SC", "Start forming SC", "Start following SC") -> (w253:bool[])
    n105 = Insert Into Array(array=w264, new element #1=w263, new element #2=w262, new element #3=w261, new element #4=w253) -> (w260:bool[])  [unwired: 1 in]
    n106 = Search 1D Array(1D array=w260, element=TRUE) -> (index of element=w279:i32)  [unwired: 1 in]
    n107 = To Unsigned Byte Integer(number=w279) -> (unsigned 8bit integer=w255:u8)
    n108 = case shown="20" w255 {
      tunnel: [u32 0 ("identifier") u32 0 ("identifier") u32 0 ("identifier") u32 0 ("identifier") u32 0 ("identifier") u32 3 ("identifier") u32 3 ("identifier") u32 3 ("identifier") u32 3 ("identifier") u32 3 ("identifier") u32 6 ("identifier") u32 6 ("identifier") u32 6 ("identifier") u32 6 ("identifier") u32 6 ("identifier") u32 9 ("identifier") u32 9 ("identifier") u32 9 ("identifier") u32 9 ("identifier") u32 9 ("identifier") u32 18 ("identifier") u32 18 ("identifier") u32 18 ("identifier") u32 18 ("identifier") u32 18 ("identifier") u32 18 ("identifier") _] -> w289
      tunnel: [TRUE TRUE w324 w338 w355 TRUE TRUE w396 w410 w427 TRUE TRUE w468 w482 w499 TRUE TRUE w540 w554 w571 TRUE w599 w621 w649 w670 w683 FALSE] -> w287
      tunnel: [w300 w312 w329 w345 w359 w372 w384 w401 w417 w431 w444 w456 w473 w489 w503 w516 w528 w545 w561 w575 w588 w615 w636 w663 w674 w690 _] -> w254
      frame 0 {
        w301 = u16 0 ("element")
        # "0x000"
        # "ErrorAck"
        n109 = local write "ErrAck 1"(FALSE ("SEND sp")) -> ()
        n110 = Split Number(x=u16 1) -> (hi(x)=w298:u8, lo(x)=w297:u8)
        n111 = Split Number(x=w301) -> (hi(x)=w307:u8, lo(x)=w306:u8)
        n112 = Split Number(x=w301) -> (hi(x)=w305:u8, lo(x)=w304:u8)
        n113 = Split Number(x=w301) -> (hi(x)=w303:u8, lo(x)=w302:u8)
        n114 = Build Array(w297, w298, w307, w306, w305, w304, w303, w302) -> (w300:u8[])
      }
      frame 1 {
        w311 = u16 0 ("element")
        # "0x000"
        # "shutdown"
        n115 = local write "Shutdwn 1"(FALSE ("SEND sp")) -> ()
        n116 = Split Number(x=w311) -> (hi(x)=w320:u8, lo(x)=w319:u8)
        n117 = Split Number(x=w311) -> (hi(x)=w318:u8, lo(x)=w317:u8)
        n118 = Split Number(x=w311) -> (hi(x)=w316:u8, lo(x)=w315:u8)
        n119 = Split Number(x=w311) -> (hi(x)=w314:u8, lo(x)=w313:u8)
        n120 = Build Array(w320, w319, w318, w317, w316, w315, w314, w313) -> (w312:u8[])
      }
      frame 2 {
        w330 = u16 0 ("element")
        # "0x000"
        # "DC link OK"
        n121 = local write "DCLinkOK 1"(FALSE ("SEND sp")) -> ()
        n122 = Split Number(x=u16 4) -> (hi(x)=w326:u8, lo(x)=w325:u8)
        n123 = Split Number(x=w330) -> (hi(x)=w336:u8, lo(x)=w335:u8)
        n124 = Split Number(x=w330) -> (hi(x)=w334:u8, lo(x)=w333:u8)
        n125 = Split Number(x=w330) -> (hi(x)=w332:u8, lo(x)=w331:u8)
        n126 = local read "Ready 1"() -> (w324:bool)
        n127 = Build Array(w325, w326, w336, w335, w334, w333, w332, w331) -> (w329:u8[])
      }
      frame 3 {
        w346 = u16 0 ("element")
        # "0x000"
        # "Power enable"
        n128 = call "Pdc_lim.vi"("IN Vdc"="P 1") -> ("OUT Vdc"=w351:dbl)  [unwired: 10 in]
        n129 = local write "PowerEnable 1"(FALSE ("SEND sp")) -> ()
        n130 = To Unsigned Word Integer(number=w351) -> (unsigned 16bit integer=w344:u16)
        n131 = Split Number(x=u16 14) -> (hi(x)=w342:u8, lo(x)=w341:u8)
        n132 = Split Number(x=w344) -> (hi(x)=w339:u8, lo(x)=w340:u8)
        n133 = Split Number(x=w346) -> (hi(x)=w350:u8, lo(x)=w349:u8)
        n134 = Split Number(x=w346) -> (hi(x)=w348:u8, lo(x)=w347:u8)
        n135 = Build Array(w341, w342, w340, w339, w350, w349, w348, w347) -> (w345:u8[])
        n136 = local read "Ready 1"() -> (w338:bool)
      }
      frame 4 {
        w360 = u16 0 ("element")
        # "0x000"
        # "Enable PR"
        n137 = local write "EnablePR 1"(FALSE ("SEND sp")) -> ()
        n138 = Split Number(x=u16 2) -> (hi(x)=w357:u8, lo(x)=w356:u8)
        n139 = Split Number(x=w360) -> (hi(x)=w366:u8, lo(x)=w365:u8)
        n140 = Split Number(x=w360) -> (hi(x)=w364:u8, lo(x)=w363:u8)
        n141 = Split Number(x=w360) -> (hi(x)=w362:u8, lo(x)=w361:u8)
        n142 = local read "OFF 1"() -> (w355:bool)
        n143 = Build Array(w356, w357, w366, w365, w364, w363, w362, w361) -> (w359:u8[])
      }
      frame 5 {
        w373 = u16 0 ("element")
        # "0x003"
        # "ErrorAck"
        n144 = local write "ErrAck 2"(FALSE ("SEND sp")) -> ()
        n145 = Split Number(x=u16 1) -> (hi(x)=w370:u8, lo(x)=w369:u8)
        n146 = Split Number(x=w373) -> (hi(x)=w379:u8, lo(x)=w378:u8)
        n147 = Split Number(x=w373) -> (hi(x)=w377:u8, lo(x)=w376:u8)
        n148 = Split Number(x=w373) -> (hi(x)=w375:u8, lo(x)=w374:u8)
        n149 = Build Array(w369, w370, w379, w378, w377, w376, w375, w374) -> (w372:u8[])
      }
      frame 6 {
        w383 = u16 0 ("element")
        # "0x003"
        # "shutdown"
        n150 = local write "Shutdwn 2"(FALSE ("SEND sp")) -> ()
        n151 = Split Number(x=w383) -> (hi(x)=w392:u8, lo(x)=w391:u8)
        n152 = Split Number(x=w383) -> (hi(x)=w390:u8, lo(x)=w389:u8)
        n153 = Split Number(x=w383) -> (hi(x)=w388:u8, lo(x)=w387:u8)
        n154 = Split Number(x=w383) -> (hi(x)=w386:u8, lo(x)=w385:u8)
        n155 = Build Array(w392, w391, w390, w389, w388, w387, w386, w385) -> (w384:u8[])
      }
      frame 7 {
        w402 = u16 0 ("element")
        # "0x003"
        # "DC link OK"
        n156 = local write "DCLinkOK 2"(FALSE ("SEND sp")) -> ()
        n157 = Split Number(x=u16 4) -> (hi(x)=w398:u8, lo(x)=w397:u8)
        n158 = Split Number(x=w402) -> (hi(x)=w408:u8, lo(x)=w407:u8)
        n159 = Split Number(x=w402) -> (hi(x)=w406:u8, lo(x)=w405:u8)
        n160 = Split Number(x=w402) -> (hi(x)=w404:u8, lo(x)=w403:u8)
        n161 = local read "Ready 2"() -> (w396:bool)
        n162 = Build Array(w397, w398, w408, w407, w406, w405, w404, w403) -> (w401:u8[])
      }
      frame 8 {
        w418 = u16 0 ("element")
        # "0x003"
        # "Power enable"
        n163 = call "Pdc_lim.vi"("IN Vdc"="P 2") -> ("OUT Vdc"=w423:dbl)  [unwired: 10 in]
        n164 = local write "PowerEnable 2"(FALSE ("SEND sp")) -> ()
        n165 = To Unsigned Word Integer(number=w423) -> (unsigned 16bit integer=w416:u16)
        n166 = Split Number(x=u16 14) -> (hi(x)=w414:u8, lo(x)=w413:u8)
        n167 = Split Number(x=w416) -> (hi(x)=w411:u8, lo(x)=w412:u8)
        n168 = Split Number(x=w418) -> (hi(x)=w422:u8, lo(x)=w421:u8)
        n169 = Split Number(x=w418) -> (hi(x)=w420:u8, lo(x)=w419:u8)
        n170 = Build Array(w413, w414, w412, w411, w422, w421, w420, w419) -> (w417:u8[])
        n171 = local read "Ready 2"() -> (w410:bool)
      }
      frame 9 {
        w432 = u16 0 ("element")
        # "0x003"
        # "Enable PR"
        n172 = local write "EnablePR 2"(FALSE ("SEND sp")) -> ()
        n173 = Split Number(x=u16 2) -> (hi(x)=w429:u8, lo(x)=w428:u8)
        n174 = Split Number(x=w432) -> (hi(x)=w438:u8, lo(x)=w437:u8)
        n175 = Split Number(x=w432) -> (hi(x)=w436:u8, lo(x)=w435:u8)
        n176 = Split Number(x=w432) -> (hi(x)=w434:u8, lo(x)=w433:u8)
        n177 = local read "OFF 2"() -> (w427:bool)
        n178 = Build Array(w428, w429, w438, w437, w436, w435, w434, w433) -> (w431:u8[])
      }
      frame 10 {
        w445 = u16 0 ("element")
        # "0x006"
        # "ErrorAck"
        n179 = local write "ErrAck 3"(FALSE ("SEND sp")) -> ()
        n180 = Split Number(x=u16 1) -> (hi(x)=w442:u8, lo(x)=w441:u8)
        n181 = Split Number(x=w445) -> (hi(x)=w451:u8, lo(x)=w450:u8)
        n182 = Split Number(x=w445) -> (hi(x)=w449:u8, lo(x)=w448:u8)
        n183 = Split Number(x=w445) -> (hi(x)=w447:u8, lo(x)=w446:u8)
        n184 = Build Array(w441, w442, w451, w450, w449, w448, w447, w446) -> (w444:u8[])
      }
      frame 11 {
        w455 = u16 0 ("element")
        # "0x006"
        # "shutdown"
        n185 = local write "Shutdwn 3"(FALSE ("SEND sp")) -> ()
        n186 = Split Number(x=w455) -> (hi(x)=w464:u8, lo(x)=w463:u8)
        n187 = Split Number(x=w455) -> (hi(x)=w462:u8, lo(x)=w461:u8)
        n188 = Split Number(x=w455) -> (hi(x)=w460:u8, lo(x)=w459:u8)
        n189 = Split Number(x=w455) -> (hi(x)=w458:u8, lo(x)=w457:u8)
        n190 = Build Array(w464, w463, w462, w461, w460, w459, w458, w457) -> (w456:u8[])
      }
      frame 12 {
        w474 = u16 0 ("element")
        # "0x006"
        # "DC link OK"
        n191 = local write "DCLinkOK  3"(FALSE ("SEND sp")) -> ()
        n192 = Split Number(x=u16 4) -> (hi(x)=w470:u8, lo(x)=w469:u8)
        n193 = Split Number(x=w474) -> (hi(x)=w480:u8, lo(x)=w479:u8)
        n194 = Split Number(x=w474) -> (hi(x)=w478:u8, lo(x)=w477:u8)
        n195 = Split Number(x=w474) -> (hi(x)=w476:u8, lo(x)=w475:u8)
        n196 = local read "Ready 3"() -> (w468:bool)
        n197 = Build Array(w469, w470, w480, w479, w478, w477, w476, w475) -> (w473:u8[])
      }
      frame 13 {
        w490 = u16 0 ("element")
        # "0x006"
        # "Power enable"
        n198 = call "Pdc_lim.vi"("IN Vdc"="P 3") -> ("OUT Vdc"=w495:dbl)  [unwired: 10 in]
        n199 = local write "PowerEnable 3"(FALSE ("SEND sp")) -> ()
        n200 = To Unsigned Word Integer(number=w495) -> (unsigned 16bit integer=w488:u16)
        n201 = Split Number(x=u16 14) -> (hi(x)=w486:u8, lo(x)=w485:u8)
        n202 = Split Number(x=w488) -> (hi(x)=w483:u8, lo(x)=w484:u8)
        n203 = Split Number(x=w490) -> (hi(x)=w494:u8, lo(x)=w493:u8)
        n204 = Split Number(x=w490) -> (hi(x)=w492:u8, lo(x)=w491:u8)
        n205 = Build Array(w485, w486, w484, w483, w494, w493, w492, w491) -> (w489:u8[])
        n206 = local read "Ready 3"() -> (w482:bool)
      }
      frame 14 {
        w504 = u16 0 ("element")
        # "0x006"
        # "Enable PR"
        n207 = local write "EnablePR 3"(FALSE ("SEND sp")) -> ()
        n208 = Split Number(x=u16 2) -> (hi(x)=w501:u8, lo(x)=w500:u8)
        n209 = Split Number(x=w504) -> (hi(x)=w510:u8, lo(x)=w509:u8)
        n210 = Split Number(x=w504) -> (hi(x)=w508:u8, lo(x)=w507:u8)
        n211 = Split Number(x=w504) -> (hi(x)=w506:u8, lo(x)=w505:u8)
        n212 = local read "OFF 3"() -> (w499:bool)
        n213 = Build Array(w500, w501, w510, w509, w508, w507, w506, w505) -> (w503:u8[])
      }
      frame 15 {
        w517 = u16 0 ("element")
        # "0x009"
        # "ErrorAck"
        n214 = local write "ErrAck 4"(FALSE ("SEND sp")) -> ()
        n215 = Split Number(x=u16 1) -> (hi(x)=w514:u8, lo(x)=w513:u8)
        n216 = Split Number(x=w517) -> (hi(x)=w523:u8, lo(x)=w522:u8)
        n217 = Split Number(x=w517) -> (hi(x)=w521:u8, lo(x)=w520:u8)
        n218 = Split Number(x=w517) -> (hi(x)=w519:u8, lo(x)=w518:u8)
        n219 = Build Array(w513, w514, w523, w522, w521, w520, w519, w518) -> (w516:u8[])
      }
      frame 16 {
        w527 = u16 0 ("element")
        # "0x009"
        # "shutdown"
        n220 = local write "Shutdwn 4"(FALSE ("SEND sp")) -> ()
        n221 = Split Number(x=w527) -> (hi(x)=w536:u8, lo(x)=w535:u8)
        n222 = Split Number(x=w527) -> (hi(x)=w534:u8, lo(x)=w533:u8)
        n223 = Split Number(x=w527) -> (hi(x)=w532:u8, lo(x)=w531:u8)
        n224 = Split Number(x=w527) -> (hi(x)=w530:u8, lo(x)=w529:u8)
        n225 = Build Array(w536, w535, w534, w533, w532, w531, w530, w529) -> (w528:u8[])
      }
      frame 17 {
        w546 = u16 0 ("element")
        # "0x009"
        # "DC link OK"
        n226 = local write "DCLinkOK  4"(FALSE ("SEND sp")) -> ()
        n227 = Split Number(x=u16 4) -> (hi(x)=w542:u8, lo(x)=w541:u8)
        n228 = Split Number(x=w546) -> (hi(x)=w552:u8, lo(x)=w551:u8)
        n229 = Split Number(x=w546) -> (hi(x)=w550:u8, lo(x)=w549:u8)
        n230 = Split Number(x=w546) -> (hi(x)=w548:u8, lo(x)=w547:u8)
        n231 = local read "Ready 4"() -> (w540:bool)
        n232 = Build Array(w541, w542, w552, w551, w550, w549, w548, w547) -> (w545:u8[])
      }
      frame 18 {
        w562 = u16 0 ("element")
        # "0x009"
        # "Power enable"
        n233 = call "Pdc_lim.vi"("IN Vdc"="P 4") -> ("OUT Vdc"=w567:dbl)  [unwired: 10 in]
        n234 = local write "PowerEnable 4"(FALSE ("SEND sp")) -> ()
        n235 = To Unsigned Word Integer(number=w567) -> (unsigned 16bit integer=w560:u16)
        n236 = Split Number(x=u16 14) -> (hi(x)=w558:u8, lo(x)=w557:u8)
        n237 = Split Number(x=w560) -> (hi(x)=w555:u8, lo(x)=w556:u8)
        n238 = Split Number(x=w562) -> (hi(x)=w566:u8, lo(x)=w565:u8)
        n239 = Split Number(x=w562) -> (hi(x)=w564:u8, lo(x)=w563:u8)
        n240 = Build Array(w557, w558, w556, w555, w566, w565, w564, w563) -> (w561:u8[])
        n241 = local read "Ready 4"() -> (w554:bool)
      }
      frame 19 {
        w576 = u16 0 ("element")
        # "0x009"
        # "Enable PR"
        n242 = local write "EnablePR 4"(FALSE ("SEND sp")) -> ()
        n243 = Split Number(x=u16 2) -> (hi(x)=w573:u8, lo(x)=w572:u8)
        n244 = Split Number(x=w576) -> (hi(x)=w582:u8, lo(x)=w581:u8)
        n245 = Split Number(x=w576) -> (hi(x)=w580:u8, lo(x)=w579:u8)
        n246 = Split Number(x=w576) -> (hi(x)=w578:u8, lo(x)=w577:u8)
        n247 = local read "OFF 4"() -> (w571:bool)
        n248 = Build Array(w572, w573, w582, w581, w580, w579, w578, w577) -> (w575:u8[])
      }
      frame 20 {
        w589 = u16 0 ("element")
        # "SC"
        # "0x00C"
        # "shut down"
        n249 = local write "Shutdwn SC"(FALSE ("SEND sp")) -> ()
        n250 = Split Number(x=u16 20) -> (hi(x)=w586:u8, lo(x)=w585:u8)
        n251 = Split Number(x=w589) -> (hi(x)=w595:u8, lo(x)=w594:u8)
        n252 = Split Number(x=w589) -> (hi(x)=w593:u8, lo(x)=w592:u8)
        n253 = Split Number(x=w589) -> (hi(x)=w591:u8, lo(x)=w590:u8)
        n254 = Build Array(w585, w586, w595, w594, w593, w592, w591, w590) -> (w588:u8[])
      }
      frame 21 {
        # "SC"
        # "0x00C"
        # "send sp"
        n255 = call "Pdc_lim.vi"("IN Vdc"="Pdc SC") -> ("OUT Vdc"=w619:dbl)  [unwired: 10 in]
        n256 = call "V_limiter.vi"("IN Q"="Vdc SC") -> ("OUT Q"=w606:dbl)  [unwired: 10 in]
        n257 = local write "SEND sp SC"(FALSE ("SEND sp SC")) -> ()
        n258 = To Word Integer(number=w619) -> (16bit integer=w614:i16)
        n259 = To Unsigned Word Integer(number=w606) -> (unsigned 16bit integer=w605:u16)
        n260 = Split Number(x=u16 14) -> (hi(x)=w612:u8, lo(x)=w611:u8)
        n261 = Split Number(x=w614) -> (hi(x)=w609:u8, lo(x)=w610:u8)
        n262 = Split Number(x=w605) -> (hi(x)=w603:u8, lo(x)=w604:u8)
        n263 = Split Number(x=u16 0 ("element")) -> (hi(x)=w618:u8, lo(x)=w617:u8)
        n264 = Build Array(w611, w612, w610, w609, w604, w603, w618, w617) -> (w615:u8[])
        n265 = local read "Ready SC"() -> (w600:bool)
        n266 = local read "ON SC"() -> (w601:bool)
        n267 = Or(x=w601, y=w600) -> (x .or. y?=w599:bool)
      }
      frame 22 {
        # "it take on average 500ms to close the switch\n-> therefore, we wait 200ms so the converter is only following in grid connected mode for 300ms\n-> this guarentees a more smooth stransition"
        # "SC"
        # "0x00C"
        # "send sp"
        n268 = local read "Pdc SC"() -> (w624:dbl)
        n269 = local read "Vdc SC"() -> (w623:dbl)
        n270 = local write "Start forming SC"(FALSE ("SEND sp")) -> ()
        n271 = call "Pdc_lim.vi"("IN Vdc"=w624) -> ("OUT Vdc"=w640:dbl)  [unwired: 10 in]
        n272 = call "V_limiter.vi"("IN Q"=w623) -> ("OUT Q"=w629:dbl)  [unwired: 10 in]
        n273 = To Word Integer(number=w640) -> (16bit integer=w635:i16)
        n274 = To Unsigned Word Integer(number=w629) -> (unsigned 16bit integer=w628:u16)
        n275 = Split Number(x=u16 4) -> (hi(x)=w633:u8, lo(x)=w632:u8)
        n276 = Split Number(x=w635) -> (hi(x)=w630:u8, lo(x)=w631:u8)
        n277 = Split Number(x=w628) -> (hi(x)=w626:u8, lo(x)=w627:u8)
        n278 = Split Number(x=u16 0 ("element")) -> (hi(x)=w639:u8, lo(x)=w638:u8)
        n279 = Build Array(w632, w633, w631, w630, w627, w626, w639, w638) -> (w636:u8[])
        n280 = flat-sequence {
          tunnel: [w642] -> w622
          tunnel: [w646] -> w621
          tunnel: w622 -> [w646]
          frame #0 {
            n281 = local read "Ready SC"() -> (w644:bool)
            n282 = local read "ON SC"() -> (w643:bool)
            n283 = Or(x=w643, y=w644) -> (x .or. y?=w642:bool)
          }
          frame #1 {
            n284 = Wait (ms)(milliseconds to wait=u32 20) -> ()  [unwired: 1 out]
          }
        }
      }
      frame 23 {
        # "it take on average 140ms to open the switch\n-> to be sure the grid is connected before we stors following, we add a 300ms delay\n-> the converter can easily sustain 160ms in forming mode when grid connected"
        # "SC"
        # "0x00C"
        # "send sp"
        n285 = local read "Pdc SC"() -> (w651:dbl)
        n286 = local read "Vdc SC"() -> (w650:dbl)
        n287 = local write "Start following SC"(FALSE ("SEND sp")) -> ()
        n288 = call "Pdc_lim.vi"("IN Vdc"=w651) -> ("OUT Vdc"=w667:dbl)  [unwired: 10 in]
        n289 = call "V_limiter.vi"("IN Q"=w650) -> ("OUT Q"=w656:dbl)  [unwired: 10 in]
        n290 = To Word Integer(number=w667) -> (16bit integer=w662:i16)
        n291 = To Unsigned Word Integer(number=w656) -> (unsigned 16bit integer=w655:u16)
        n292 = Split Number(x=u16 3) -> (hi(x)=w660:u8, lo(x)=w659:u8)
        n293 = Split Number(x=w662) -> (hi(x)=w657:u8, lo(x)=w658:u8)
        n294 = Split Number(x=w655) -> (hi(x)=w653:u8, lo(x)=w654:u8)
        n295 = Split Number(x=u16 0 ("element")) -> (hi(x)=w666:u8, lo(x)=w665:u8)
        n296 = Build Array(w659, w660, w658, w657, w654, w653, w666, w665) -> (w663:u8[])
        n297 = local read "Ready SC"() -> (w648:bool)
        n298 = local read "ON SC"() -> (w647:bool)
        n299 = Or(x=w647, y=w648) -> (x .or. y?=w649:bool)
      }
      frame 25 {
        w675 = u16 0 ("element")
        # "SC"
        # "0x00C"
        # "start forming"
        n300 = local write "SEND sp SC"(TRUE ("SEND sp SC")) -> ()
        n301 = Split Number(x=u16 4) -> (hi(x)=w672:u8, lo(x)=w671:u8)
        n302 = Split Number(x=w675) -> (hi(x)=w681:u8, lo(x)=w680:u8)
        n303 = Split Number(x=w675) -> (hi(x)=w679:u8, lo(x)=w678:u8)
        n304 = Split Number(x=w675) -> (hi(x)=w677:u8, lo(x)=w676:u8)
        n305 = local read "ON SC"() -> (w670:bool)
        n306 = Build Array(w671, w672, w681, w680, w679, w678, w677, w676) -> (w674:u8[])
      }
      frame 26 {
        w691 = u16 0 ("element")
        # "SC"
        # "0x00C"
        # "start following"
        n307 = local write "SEND sp SC"(TRUE ("SEND sp SC")) -> ()
        n308 = local write "Start following SC"(FALSE ("SEND sp")) -> ()
        n309 = Split Number(x=u16 3) -> (hi(x)=w688:u8, lo(x)=w687:u8)
        n310 = local read "Ready SC"() -> (w685:bool)
        n311 = Split Number(x=w691) -> (hi(x)=w697:u8, lo(x)=w696:u8)
        n312 = Split Number(x=w691) -> (hi(x)=w695:u8, lo(x)=w694:u8)
        n313 = Split Number(x=w691) -> (hi(x)=w693:u8, lo(x)=w692:u8)
        n314 = local read "ON SC"() -> (w684:bool)
        n315 = Build Array(w687, w688, w697, w696, w695, w694, w693, w692) -> (w690:u8[])
        n316 = Or(x=w684, y=w685) -> (x .or. y?=w683:bool)
      }
      frame 100, Default {
      }
    }
    n317 = Get Date/Time In Seconds() -> (seconds since 1Jan1904=w252:timestamp)
    n318 = Bundle By Name(cluster=T4 {"timestamp"=timestamp(0 s since 1904-01-01), "payload"=[], "identifier"=0, "type"=0, "extended?"=FALSE, "echo?"=FALSE} ("CAN frame 3"), "payload"=w254, "identifier"=w289, "timestamp"=w252) -> (w286:T4)
    n319 = local read "main stop"() -> (w283:bool)
    n320 = case shown="True" w287 {
      tunnel: w286 -> [w293 _]
      tunnel: w285 -> [w295 _]
      tunnel: [w294 _] -> w284
      frame True {
        n321 = Build Array(w293) -> (w296:T4[])
        n322 = call-poly <vilib>:"XNET Write.vi"("session in"=w295, "data"=w296) -> ("session out"=w294:refnum<k21>)  [unwired: 12 in, 1 out]
        "CAN OUT" <- w293
      }
      frame False {
      }
    }
    n323 = node-c288() -> ()  [unwired: 1 in, 1 out]
  }
  n324 = timed-loop {
    timing: w85 -> [_]
    timing-out: [_] -> w84
    tunnel: w83 -> [w706]
    tunnel: [w710] -> w89
    tunnel: [FALSE ("stop CAN")] -> w87
    shift-right: [w704] -> _
    shift-left: T3 {"V_PV1"=0.0, "V_CAP1"=0.0, "V_PV2"=0.0, "V_CAP2"=0.0, "V_grid2"=0.0, "V_PV3"=0.0, "V_CAP3"=0.0, "V_grid3"=0.0, "V_PV4"=0.0, "V_CAP4"=0.0, "V_grid4"=0.0, "V_grid1"=0.0, "P1"=0.0, "P2"=0.0, "P3"=0.0, "P4"=0.0} ("measurements 2") -> [w705]
    shift-right: [w701] -> _
    shift-left: T2 {"V_SC"=0.0, "V_CAP"=0.0, "V_grid"=0.0, "P"=0.0, "SOC"=0.0} ("measurements SuperCap") -> [w702]
    stop <- w709 stop-if-true
    # "READ CAN FROM CONVERTER"
    n325 = node-c288() -> ()  [unwired: 1 in, 1 out]
    n326 = Get Date/Time In Seconds() -> (seconds since 1Jan1904=→"current time":timestamp)
    n327 = local write "CAN with Conv"(TRUE) -> ()
    n328 = call-poly <vilib>:"XNET Read.vi"("session in"=w706) -> ("session out"=w710:refnum<k21>, "data"=w711:T4[])  [unwired: 11 in, 2 out]
    n329 = for {
      tunnel: w711 -> [w716] mode=indexing
      shift-right: [w714] -> w704
      shift-left: w705 -> [w715]
      shift-right: [w712] -> w701
      shift-left: w702 -> [w713]
      n330 = Unbundle By Name(w716) -> ("identifier"=w718:u32, "payload"=w717:u8[])
      n331 = case shown="1" w718 {
        tunnel: w717 -> [_ w727 w734 w741 w748 w774 w778 w805 w832 w859 w897]
        tunnel: w715 -> [w719 w725 w732 w739 w746 w770 w779 w806 w833 w860 w893]
        tunnel: [w719 w726 w733 w740 w747 w770 w780 w807 w834 w861 w893] -> w714
        tunnel: w713 -> [w720 w721 w728 w735 w742 w772 w775 w802 w829 w856 w895]
        tunnel: [w720 w721 w728 w735 w742 w771 w775 w802 w829 w856 w894] -> w712
        frame 0, Default {
        }
        frame 1 {
          # "0x001"
          # "P"
          n332 = call "U8arrayToMeasurement.vi"("payload"=w727) -> ("Meas 4"=w722:dbl, "Meas 1"=w723:dbl, "Meas 2"=w724:dbl)  [unwired: 4 in, 1 out]
          "V slider 28" <- w723
          "V slider 27" <- w722
          n333 = Bundle By Name(cluster=w725, "V_CAP1"=w724, "V_PV1"=w723, "V_grid1"=w722) -> (w726:T3)
        }
        frame 4 {
          # "0x004"
          # "P"
          n334 = call "U8arrayToMeasurement.vi"("payload"=w734) -> ("Meas 4"=w729:dbl, "Meas 1"=w730:dbl, "Meas 2"=w731:dbl)  [unwired: 4 in, 1 out]
          "V slider 26" <- w730
          "V slider 25" <- w729
          n335 = Bundle By Name(cluster=w732, "V_CAP2"=w731, "V_PV2"=w730, "V_grid2"=w729) -> (w733:T3)
        }
        frame 7 {
          # "0x007"
          # "P"
          n336 = call "U8arrayToMeasurement.vi"("payload"=w741) -> ("Meas 4"=w736:dbl, "Meas 1"=w737:dbl, "Meas 2"=w738:dbl)  [unwired: 4 in, 1 out]
          "V slider 24" <- w737
          "V slider 23" <- w736
          n337 = Bundle By Name(cluster=w739, "V_CAP3"=w738, "V_PV3"=w737, "V_grid3"=w736) -> (w740:T3)
        }
        frame 10 {
          # "0x00A"
          # "P"
          n338 = call "U8arrayToMeasurement.vi"("payload"=w748) -> ("Meas 4"=w744:dbl, "Meas 1"=w743:dbl, "Meas 2"=w745:dbl)  [unwired: 4 in, 1 out]
          "V slider 21" <- w744
          "V slider 22" <- w743
          n339 = Bundle By Name(cluster=w746, "V_CAP4"=w745, "V_PV4"=w743, "V_grid4"=w744) -> (w747:T3)
        }
        frame 14 {
          w760 = i16 -2 ("n")
          w761 = 16.0 ("Meas 1")
          # "Vmax"
          # "Vmin"
          # "F"
          # "0x00E"
          # "P"
          n340 = call "U8arrayToMeasurement.vi"("payload"=w774) -> ("Meas 4"=w773:dbl, "Meas 1"=w750:dbl, "Meas 2"=w749:dbl)  [unwired: 4 in, 1 out]
          "V slider 30" <- w750
          "V slider 29" <- w749
          n341 = Square(x=150.0 ("Meas 1")) -> (x^2=w766:dbl)
          n342 = Square(x=300.0 ("Meas 1")) -> (x^2=w767:dbl)
          n343 = Square(x=w750) -> (x^2=w763:dbl)
          n344 = Multiply(x=w766, y=w761) -> (x*y=w765:dbl)
          n345 = Multiply(x=w767, y=w761) -> (x*y=w764:dbl)
          n346 = Multiply(x=w763, y=w761) -> (x*y=w762:dbl)
          n347 = Scale By Power Of 2(n=w760, x=w765) -> (x*2^n=w757:dbl)
          n348 = Scale By Power Of 2(n=w760, x=w762) -> (x*2^n=w759:dbl)
          n349 = Scale By Power Of 2(n=w760, x=w764) -> (x*2^n=w758:dbl)
          n350 = Subtract(x=w759, y=w757) -> (x-y=w756:dbl)
          n351 = Subtract(x=w758, y=w757) -> (x-y=w755:dbl)
          n352 = Divide(x=w756, y=w755) -> (x/y=w753:dbl)
          n353 = Multiply(x=w753, y=100.0) -> (x*y=w752:dbl)
          n354 = Round To Nearest(number=w752) -> (nearest integer value=w754:dbl)
          "V slider 31" <- w754
          n355 = Bundle By Name(cluster=w772, "V_CAP"=w749, "V_SC"=w750, "V_grid"=w773, "SOC"=w754) -> (w771:T2)
        }
        frame 2 {
          # "0x002"
          n356 = call "U8arrayToMeasurement2.vi"("payload"=w778) -> ("Meas 2"=w776:dbl, "uint16"=w777:u16)  [unwired: 4 in, 2 out]
          "kW" <- w776
          "state 1" <- w777
          n357 = case shown="1" w777 {
            frame 3 {
              # "idle"
              n358 = local write "ON 1"(FALSE ("ON 1")) -> ()
              n359 = local write "Ready 1"(TRUE ("Ready 1")) -> ()
              n360 = local write "OFF 1"(FALSE ("OFF 1")) -> ()
            }
            frame 4 {
              # "mppt"
              n361 = local write "ON 1"(FALSE ("ON 1")) -> ()
              n362 = local write "Ready 1"(TRUE ("Ready 1")) -> ()
              n363 = local write "OFF 1"(FALSE ("OFF 1")) -> ()
            }
            frame 5 {
              # "mppt"
              n364 = local write "ON 1"(TRUE ("ON 1")) -> ()
              n365 = local write "Ready 1"(FALSE ("Ready 1")) -> ()
              n366 = local write "OFF 1"(FALSE ("OFF 1")) -> ()
            }
            frame 0 {
              # "to precharge"
              n367 = local write "ON 1"(FALSE ("ON 1")) -> ()
              n368 = local write "Ready 1"(FALSE ("Ready 1")) -> ()
              n369 = local write "OFF 1"(TRUE ("OFF 1")) -> ()
            }
            frame 6, Default {
              # "to precharge"
              n370 = local write "ON 1"(FALSE ("ON 1")) -> ()
              n371 = local write "Ready 1"(FALSE ("Ready 1")) -> ()
              n372 = local write "OFF 1"(FALSE ("OFF 1")) -> ()
            }
            frame 1 {
              # "precharge"
              n373 = local write "ON 1"(FALSE ("ON 1")) -> ()
              n374 = local write "Ready 1"(FALSE ("Ready 1")) -> ()
              n375 = local write "OFF 1"(TRUE ("OFF 1")) -> ()
            }
            frame 2 {
              # "standby"
              n376 = local write "ON 1"(FALSE ("ON 1")) -> ()
              n377 = local write "Ready 1"(TRUE ("Ready 1")) -> ()
              n378 = local write "OFF 1"(FALSE ("OFF 1")) -> ()
            }
          }
          n379 = Bundle By Name(cluster=w779, "P1"=w776) -> (w780:T3)
        }
        frame 5 {
          # "0x005"
          n380 = call "U8arrayToMeasurement2.vi"("payload"=w805) -> ("Meas 2"=w803:dbl, "uint16"=w804:u16)  [unwired: 4 in, 2 out]
          "state 2" <- w804
          "kW" <- w803
          n381 = case shown="6, Default" w804 {
            frame 3 {
              # "idle"
              n382 = local write "ON 2"(FALSE ("ON 1")) -> ()
              n383 = local write "Ready 2"(TRUE ("Ready 1")) -> ()
              n384 = local write "OFF 2"(FALSE ("OFF 1")) -> ()
            }
            frame 4 {
              # "mppt"
              n385 = local write "ON 2"(FALSE ("ON 1")) -> ()
              n386 = local write "Ready 2"(TRUE ("Ready 1")) -> ()
              n387 = local write "OFF 2"(FALSE ("OFF 1")) -> ()
            }
            frame 5 {
              # "mppt"
              n388 = local write "ON 2"(TRUE ("ON 1")) -> ()
              n389 = local write "Ready 2"(FALSE ("Ready 1")) -> ()
              n390 = local write "OFF 2"(FALSE ("OFF 1")) -> ()
            }
            frame 0 {
              # "to precharge"
              n391 = local write "ON 2"(FALSE ("ON 1")) -> ()
              n392 = local write "Ready 2"(FALSE ("Ready 1")) -> ()
              n393 = local write "OFF 2"(TRUE ("OFF 1")) -> ()
            }
            frame 6, Default {
              # "to precharge"
              n394 = local write "ON 2"(FALSE ("ON 1")) -> ()
              n395 = local write "Ready 2"(FALSE ("Ready 1")) -> ()
              n396 = local write "OFF 2"(FALSE ("OFF 1")) -> ()
            }
            frame 1 {
              # "precharge"
              n397 = local write "ON 2"(FALSE ("ON 1")) -> ()
              n398 = local write "Ready 2"(FALSE ("Ready 1")) -> ()
              n399 = local write "OFF 2"(TRUE ("OFF 1")) -> ()
            }
            frame 2 {
              # "standby"
              n400 = local write "ON 2"(FALSE ("ON 1")) -> ()
              n401 = local write "Ready 2"(TRUE ("Ready 1")) -> ()
              n402 = local write "OFF 2"(FALSE ("OFF 1")) -> ()
            }
          }
          n403 = Bundle By Name(cluster=w806, "P2"=w803) -> (w807:T3)
        }
        frame 8 {
          # "0x008"
          n404 = call "U8arrayToMeasurement2.vi"("payload"=w832) -> ("Meas 2"=w830:dbl, "uint16"=w831:u16)  [unwired: 4 in, 2 out]
          "state 3" <- w831
          "kW" <- w830
          n405 = case shown="2" w831 {
            frame 3 {
              # "idle"
              n406 = local write "ON 3"(FALSE ("ON 1")) -> ()
              n407 = local write "Ready 3"(TRUE ("Ready 1")) -> ()
              n408 = local write "OFF 3"(FALSE ("OFF 1")) -> ()
            }
            frame 4 {
              # "mppt"
              n409 = local write "ON 3"(FALSE ("ON 1")) -> ()
              n410 = local write "Ready 3"(TRUE ("Ready 1")) -> ()
              n411 = local write "OFF 3"(FALSE ("OFF 1")) -> ()
            }
            frame 5 {
              # "mppt"
              n412 = local write "ON 3"(TRUE ("ON 1")) -> ()
              n413 = local write "Ready 3"(FALSE ("Ready 1")) -> ()
              n414 = local write "OFF 3"(FALSE ("OFF 1")) -> ()
            }
            frame 0 {
              # "to precharge"
              n415 = local write "ON 3"(FALSE ("ON 1")) -> ()
              n416 = local write "Ready 3"(FALSE ("Ready 1")) -> ()
              n417 = local write "OFF 3"(TRUE ("OFF 1")) -> ()
            }
            frame 6, Default {
              # "to precharge"
              n418 = local write "ON 3"(FALSE ("ON 1")) -> ()
              n419 = local write "Ready 3"(FALSE ("Ready 1")) -> ()
              n420 = local write "OFF 3"(FALSE ("OFF 1")) -> ()
            }
            frame 1 {
              # "precharge"
              n421 = local write "ON 3"(FALSE ("ON 1")) -> ()
              n422 = local write "Ready 3"(FALSE ("Ready 1")) -> ()
              n423 = local write "OFF 3"(TRUE ("OFF 1")) -> ()
            }
            frame 2 {
              # "standby"
              n424 = local write "ON 3"(FALSE ("ON 1")) -> ()
              n425 = local write "Ready 3"(TRUE ("Ready 1")) -> ()
              n426 = local write "OFF 3"(FALSE ("OFF 1")) -> ()
            }
          }
          n427 = Bundle By Name(cluster=w833, "P3"=w830) -> (w834:T3)
        }
        frame 11 {
          # "0x00B"
          n428 = call "U8arrayToMeasurement2.vi"("payload"=w859) -> ("Meas 2"=w857:dbl, "uint16"=w858:u16)  [unwired: 4 in, 2 out]
          "state 4" <- w858
          "kW" <- w857
          n429 = case shown="5" w858 {
            frame 3 {
              # "idle"
              n430 = local write "ON 4"(FALSE ("ON 1")) -> ()
              n431 = local write "Ready 4"(TRUE ("Ready 1")) -> ()
              n432 = local write "OFF 4"(FALSE ("OFF 1")) -> ()
            }
            frame 4 {
              # "mppt"
              n433 = local write "ON 4"(FALSE ("ON 1")) -> ()
              n434 = local write "Ready 4"(TRUE ("Ready 1")) -> ()
              n435 = local write "OFF 4"(FALSE ("OFF 1")) -> ()
            }
            frame 5 {
              # "mppt"
              n436 = local write "ON 4"(TRUE ("ON 1")) -> ()
              n437 = local write "Ready 4"(FALSE ("Ready 1")) -> ()
              n438 = local write "OFF 4"(FALSE ("OFF 1")) -> ()
            }
            frame 0 {
              # "to precharge"
              n439 = local write "ON 4"(FALSE ("ON 1")) -> ()
              n440 = local write "Ready 4"(FALSE ("Ready 1")) -> ()
              n441 = local write "OFF 4"(TRUE ("OFF 1")) -> ()
            }
            frame 6, Default {
              # "to precharge"
              n442 = local write "ON 4"(FALSE ("ON 1")) -> ()
              n443 = local write "Ready 4"(FALSE ("Ready 1")) -> ()
              n444 = local write "OFF 4"(FALSE ("OFF 1")) -> ()
            }
            frame 1 {
              # "precharge"
              n445 = local write "ON 4"(FALSE ("ON 1")) -> ()
              n446 = local write "Ready 4"(FALSE ("Ready 1")) -> ()
              n447 = local write "OFF 4"(TRUE ("OFF 1")) -> ()
            }
            frame 2 {
              # "standby"
              n448 = local write "ON 4"(FALSE ("ON 1")) -> ()
              n449 = local write "Ready 4"(TRUE ("Ready 1")) -> ()
              n450 = local write "OFF 4"(FALSE ("OFF 1")) -> ()
            }
          }
          n451 = Bundle By Name(cluster=w860, "P4"=w857) -> (w861:T3)
        }
        frame 15 {
          # "0x00F"
          n452 = call "U8arrayToMeasurement2.vi"("payload"=w897) -> ("Meas 2"=w896:dbl, "uint16"=w890:u16)  [unwired: 4 in, 2 out]
          "state SC" <- w890
          "kW" <- w896
          n453 = Equal?(x=w890, y=u16 43) -> (x = y?=w887:bool)
          n454 = Equal?(x=w890, y=u16 44) -> (x = y?=w883:bool)
          "forming?" <- w883
          n455 = Equal?(x=w890, y=u16 41) -> (x = y?=w886:bool)
          n456 = Or(x=w887, y=w883) -> (x .or. y?=w892:bool)
          n457 = Compound Arithmetic op=OR(w887, w883, w886) -> (w885:bool)
          n458 = local write "Ready SC"(w886) -> ()
          n459 = Bundle By Name(cluster=w895, "P"=w896) -> (w894:T2)
          n460 = Not(x=w885) -> (.not. x?=w884:bool)
          n461 = local write "ON SC"(w892) -> ()
          n462 = local write "OFF SC"(w884) -> ()
        }
      }
      n463 = local write "measurements SuperCap"(w712) -> ()
      n464 = local write "measurements"(w714) -> ()
      "CAN IN" <- w716
    }
    n465 = local read "main stop"() -> (w709:bool)
    n466 = node-c288() -> ()  [unwired: 1 in, 1 out]
  }
  n467 = String To IP(1:w76) -> (0:w9:u32)
  n468 = while {
    tunnel: w28 -> [w904]
    tunnel: [w905] -> w23
    shift-right: [w906] -> _
    shift-left: T1 {"Synchronized?"=FALSE, "Sync Loss Count in"=0, "Current Sync Duration"=0} ("Status In") -> [w907]
    tunnel: w26 -> [w908]
    tunnel: "Loop Time" -> [w901]
    tunnel: [w903] -> w24
    stop <- w900 stop-if-true
    # "Run in parallel with \nyour other loops"
    # "Check Time Synch"
    n469 = Wait (ms)(milliseconds to wait=w901) -> ()  [unwired: 1 out]
    n470 = call "PM_Synch_Monitor.vi"("Polling Interval"=w901, "error in"=w904, "Status In"=w907, "Synch In"=w908) -> ("error out"=w905:errorcluster, "Status Out"=w906:T1, "Reference out"=w903:refnum<k15>, "Offset from TR (ns)"=→"Offset from TR (ns)":dbl)  [unwired: 3 in, 1 out]
    "Status Out" <- w906
    n471 = local read "main stop"() -> (w900:bool)
  }
  n472 = String To IP(1:w78) -> (0:w79:u32)
  n473 = UDP Open(7:w79, 9:10000 ("timeout ms (25000)"), 11:w77) -> (port=w7:refnum<k16>, 0:w6:errorcluster)  [unwired: 2 in, 1 out]
  n474 = while {
    tunnel: [w916] -> w10
    tunnel: w9 -> [w914]
    tunnel: w8 -> [w913]
    tunnel: w6 -> [w911]
    shift-right: [w910] -> w5
    shift-left: w7 -> [w912]
    stop <- w909 stop-if-true
    w915 = u32 100  # UDP refresh rate
    n475 = local read "measurements"() -> (w924:T3)
    n476 = local read "measurements SuperCap"() -> (w930:T2)
    n477 = Wait (ms)(milliseconds to wait=w915) -> ()  [unwired: 1 out]
    n478 = Get Date/Time In Seconds() -> (seconds since 1Jan1904=w919:timestamp)
    n479 = To Double Precision Float(number=w919) -> (double precision float=w923:dbl)
    n480 = local read "ON SC"() -> (w931:bool)
    n481 = local read "ON 1"() -> (w925:bool)
    n482 = local read "ON 2"() -> (w926:bool)
    n483 = local read "ON 3"() -> (w927:bool)
    n484 = local read "ON 4"() -> (w928:bool)
    n485 = Bundle By Name(cluster=T13 {"Info"={"Resource"="PV_emulator", "Problem"=FALSE, "Timestamp"=0.0}, "Data"={"Status 1"=FALSE, "Status 2"=FALSE, "measurements"={"V_PV1"=0.0, "V_CAP1"=0.0, "V_PV2"=0.0, "V_CAP2"=0.0, "V_grid2"=0.0, "V_PV3"=0.0, "V_CAP3"=0.0, "V_grid3"=0.0, "V_PV4"=0.0, "V_CAP4"=0.0, "V_grid4"=0.0, "V_grid1"=0.0, "P1"=0.0, "P2"=0.0, "P3"=0.0, "P4"=0.0}, "Status 3"=FALSE, "Status 4"=FALSE, "measurements SC"={"V_SC"=0.0, "V_CAP"=0.0, "V_grid"=0.0, "P"=0.0, "SOC"=0.0}, "Status SC"=FALSE, "Forming/Following"=FALSE, "Start forming"=FALSE, "SC references"={"Vdc"=0.0, "Pdc"=0.0}, "Start following"=FALSE}} ("Cluster"), "Info.Resource"="PV_emulator", "Info.Problem"=FALSE, "Info.Timestamp"=w923, "Data.Status 1"=w925, "Data.Status 2"=w926, "Data.Status 3"=w927, "Data.Status 4"=w928, "Data.Status SC"=w931, "Data.measurements"=w924, "Data.measurements SC"=w930) -> (w929:T13)
    n486 = Flatten To JSON(anything=w929, error in (no error)=w911) -> (JSON string=w918:string, 11:w917:errorcluster)  [unwired: 1 in]
    n487 = UDP Write(address=w914, port or service name=w913, connection ID=w912, data in=w918, 8:w917) -> (error out=w933:errorcluster, 3:w910:refnum<k16>)  [unwired: 1 in]
    n488 = local read "main stop"() -> (w909:bool)
    n489 = call <vilib>:"Clear Errors.vi"("error in (no error)"=w933, "specific error code to clear (0: all)"=56) -> ("error out"=w916:errorcluster)  [unwired: 4 in, 1 out]
  }
  n490 = node-c288(w71) -> ()  [unwired: 1 out]
  n491 = UDP Close(connection ID=w31, 8:w30) -> ()  [unwired: 2 out]
  n492 = TCP Close Connection(connection ID=w63, error in (no error)=w62) -> (error out=w64:errorcluster)  [unwired: 1 in, 1 out]
  n493 = TCP Close Connection(connection ID=w39, error in (no error)=w38) -> (error out=w42:errorcluster)  [unwired: 1 in, 1 out]
  n494 = TCP Close Connection(connection ID=w37, error in (no error)=w36) -> (error out=w41:errorcluster)  [unwired: 1 in, 1 out]
  n495 = TCP Close Connection(connection ID=w35, error in (no error)=w34) -> (error out=w40:errorcluster)  [unwired: 1 in, 1 out]
  n496 = call <vilib>:"General Error Handler.vi"("error in (no error)"=w64) -> ()  [unwired: 10 in, 5 out]
  n497 = call <vilib>:"General Error Handler.vi"("error in (no error)"=w42) -> ()  [unwired: 10 in, 5 out]
  n498 = call <vilib>:"General Error Handler.vi"("error in (no error)"=w41) -> ()  [unwired: 10 in, 5 out]
  n499 = call <vilib>:"General Error Handler.vi"("error in (no error)"=w40) -> ()  [unwired: 10 in, 5 out]
  n500 = call <instrlib>:"niSync Close.vi"("error in (no error)"=w23, "instrument handle"=w24) -> ("error out"=→"Error out":errorcluster)  [unwired: 9 in]
  n501 = while {
    stop <- w934 stop-if-true
    n502 = flat-sequence {
      tunnel: [w936] -> w935
      tunnel: w935 -> [w943]
      frame #0 {
        n503 = local read "start following SC pre"() -> (w937:bool)
        n504 = call <userlib>:"Boolean Trigger__ogtk.vi"("Boolean Input"=w937) -> ("Rising Edge"=w938:bool)  [unwired: 1 in, 1 out]
        n505 = case shown="True" w938 {
          tunnel: w937 -> [w939 w940]
          tunnel: [w939 w940] -> w936
          frame False {
          }
          frame True {
            n506 = Get Date/Time In Seconds() -> (seconds since 1Jan1904=→"time_sc":timestamp)
            n507 = Wait (ms)(milliseconds to wait=u32 650) -> ()  [unwired: 1 out]
          }
        }
      }
      frame #1 {
        n508 = local write "Start following SC"(w943) -> ()
      }
    }
    n509 = local read "main stop"() -> (w934:bool)
  }
  n510 = node-c288(w84) -> ()  [unwired: 1 out]
  n511 = node-c288(w80) -> ()  [unwired: 1 out]
  n512 = UDP Close(connection ID=w5, 8:w10) -> ()  [unwired: 2 out]
  n513 = local write "CAN with Conv"(w87) -> ()
  n514 = call <vilib>:"XNET Stop.vi"("session in"=w89) -> ()  [unwired: 13 in, 2 out]
  n515 = call <vilib>:"XNET Stop.vi"("session in"=w88) -> ()  [unwired: 13 in, 2 out]
  n516 = UDP Close(connection ID=w11, 8:w3) -> ()  [unwired: 2 out]
  "Measurements" <- w2
  "CAN with Conv" <- w2
  "Ready 1" <- w2
  "OFF 1" <- w2
  "Ready 2" <- w2
  "ON 2" <- w2
  "OFF 2" <- w2
  "Ready 4" <- w2
  "ON 4" <- w2
  "OFF 4" <- w2
  "ON 3" <- w2
  "Ready 3" <- w2
  "OFF 3" <- w2
  "ON SC" <- w2
  "OFF SC" <- w2
  "Ready SC" <- w2
